vi "Main.vi"() -> ()   [LabVIEW 2019]
uses:
  <vilib>/myRIO/Instrument Drivers/Onboard IO/DIO/typedefs/DIO Reference.ctl
  <vilib>/myRIO/Common/Instrument Driver Framework/Utilities/typedefs/myRIO Generic Hardware Reference.ctl
  <vilib>/myRIO/Common/Instrument Driver Framework/Utilities/typedefs/Hardware Version Enum.ctl
  <vilib>/myRIO/Common/Instrument Driver Framework/Utilities/typedefs/myRIO v1.0 Reference.ctl
  <vilib>/myRIO/Common/Instrument Driver Framework/Utilities/typedefs/Generic FPGA Reference.ctl
  <vilib>/myRIO/Common/Instrument Driver Framework/myRIO v1.0/DIO/typedefs/DIO Channels List.ctl
  <vilib>/myRIO/Common/Instrument Driver Framework/myRIO v1.0/DIO/typedefs/DIO Channels Enum.ctl
  <vilib>/userDefined/High Color/nirio_resource_hc.ctl
  <vilib>/myRIO/Common/Instrument Driver Framework/myRIO v1.0/Encoder/typedefs/Encoder Signal Mode.ctl
  <vilib>/myRIO/Instrument Drivers/Onboard IO/Encoder/typedefs/Encoder Reference.ctl
  <vilib>/myRIO/Common/Instrument Driver Framework/myRIO v1.0/Encoder/typedefs/Encoder Channels Enum.ctl
  <vilib>/myRIO/Common/Instrument Driver Framework/myRIO v1.0/Encoder/typedefs/Encoder Configuration v1.0.ctl
  <vilib>/myRIO/Common/Instrument Driver Framework/Utilities/vis/Is FPGA Ref Available.vi
  <vilib>/myRIO/Common/Instrument Driver Framework/myRIO v1.0/DIO/vis/myRIO v1.1 Open DIO.vi
  <vilib>/myRIO/Instrument Drivers/Onboard IO/DIO/vis/Read.vi
  <vilib>/myRIO/Common/Instrument Driver Framework/myRIO v1.0/Encoder/vis/myRIO v1.1 Open Encoder.vi
  <vilib>/myRIO/Instrument Drivers/Onboard IO/Encoder/vis/Read.vi
  <vilib>/myRIO/Instrument Drivers/Onboard IO/DIO/vis/Write.vi
  <vilib>/myRIO/Common/Instrument Driver Framework/Utilities/vis/Validate Channels.vi
  <vilib>/myRIO/Common/Instrument Driver Framework/myRIO v1.0/DIO/vis/myRIO v1.0 Reserve DIO.vi
  <vilib>/myRIO/Common/Instrument Driver Framework/myRIO v1.0/Encoder/vis/myRIO v1.0 Reserve Encoder.vi
  <vilib>/Analysis/coordinate.llb/2D Cartesian Coordinate Rotation.vi
  <vilib>/Analysis/coordinate.llb/2D Cartesian Coordinate Rotation (Scalar).vi
  <vilib>/myRIO/Common/Instrument Driver Framework/myRIO v1.0/Resource Manager/vis/myRIO v1.0 Reserve Channel List.vi
  <vilib>/myRIO/Common/Instrument Driver Framework/myRIO v1.0/DIO/vis/myRIO v1.0 Build MUX Configuration DIO.vi
  <vilib>/myRIO/Common/Instrument Driver Framework/myRIO v1.0/Encoder/vis/myRIO v1.0 Build MUX Configuration Encoder.vi
  <vilib>/myRIO/Common/Instrument Driver Framework/myRIO v1.0/Resource Manager/vis/myRIO v1.0 Reserve Channel.vi
  <vilib>/myRIO/Common/Instrument Driver Framework/myRIO v1.0/Resource Manager/vis/myRIO v1.0 Unreserve Channel.vi
  <vilib>/myRIO/Common/Instrument Driver Framework/myRIO v1.0/Resource Manager/vis/myRIO v1.0 Create Configuration List.vi
  <vilib>/myRIO/Common/Instrument Driver Framework/myRIO v1.0/Resource Manager/vis/myRIO v1.0 Build Mutex Name.vi
  Global Var.vi
  <vilib>/Instr/_visa.llb/VISA Configure Serial Port (Instr).vi
  <vilib>/addons/control/pid/pid.llb/PID (DBL).vi
  <vilib>/Utility/VariantDataType/GetNumericInfo.vi
  <vilib>/Utility/error.llb/Error Cluster From Error Code.vi
  <vilib>/myRIO/Common/Instrument Driver Framework/myRIO v1.0/myRIO v1.1 Open.vi
  <vilib>/myRIO/Common/Instrument Driver Framework/Utilities/vis/IO Manager.vi
  <vilib>/myRIO/Common/Instrument Driver Framework/Utilities/vis/Configuration Manager.vi
  <vilib>/myRIO/Common/Instrument Driver Framework/myRIO v1.0/Resource Manager/vis/myRIO v1.0 Configure IO.vi
  <vilib>/myRIO/Common/Instrument Driver Framework/myRIO v1.0/myRIO v1.0 Close.vi
  <vilib>/myRIO/Common/Instrument Driver Framework/myRIO v1.0/DIO/vis/myRIO v1.0 Write DIO.vi
  <vilib>/myRIO/Common/Instrument Driver Framework/myRIO v1.0/Encoder/vis/myRIO v1.0 Configure Encoder.vi
  <vilib>/myRIO/Common/Instrument Driver Framework/myRIO v1.0/Encoder/vis/myRIO v1.0 Read Encoder.vi
  <vilib>/myRIO/Common/Instrument Driver Framework/myRIO v1.0/DIO/vis/myRIO v1.0 Read DIO.vi
  <vilib>/myRIO/Express VI/Onboard IO/DO/DO Express VI.xnode
  <vilib>/myRIO/Instrument Drivers/Onboard IO/DIO/vis/myRIO DIO Open.xnode
  <vilib>/myRIO/Express VI/Onboard IO/Encoder/Encoder Express VI.xnode
  <vilib>/myRIO/Instrument Drivers/Onboard IO/Encoder/vis/myRIO Encoder Open.xnode
  <vilib>/myRIO/Common/Instrument Driver Framework/myRIO v1.0/Encoder/typedefs/Encoder Count Direction Enum.ctl
  <vilib>/myRIO/Express VI/Onboard IO/DI/DI Express VI.xnode
  <vilib>/myRIO/Instrument Drivers/Onboard IO/DIO/DIO.lvlib
  <vilib>/myRIO/Instrument Drivers/Onboard IO/Encoder/Encoder.lvlib
  <vilib>/addons/control/pid/NI_PID_pid.lvlib
  <vilib>/robotics/Steering/Steering Frame/NI_Robotics_Steering Frame.lvclass
panel:
  in  "Reset":bool
  out "Suctime":u32
  out "lasttime":u32
  out "time":u32
  in  "QRCodeTick":bool
  out "read buffer":string
  in  "Set Y":dbl
  in  "Set 0":bool
  out "Chart Trackline 3":cluster{"X_set":dbl, "X_en":dbl}(graph)
  in  "PID gains 6":T1={"proportional gain (Kc)"=1.5, "integral time (Ti, min)"=0.0, "derivative time (Td, min)"=0.0} {"derivative time (Td, min)" format="%.3f"; "integral time (Ti, min)" format="%.3f"; "proportional gain (Kc)" format="%.3f"}
  in  "PID gains 5":T1={"proportional gain (Kc)"=1.0, "integral time (Ti, min)"=0.0, "derivative time (Td, min)"=0.0} {"derivative time (Td, min)" format="%.3f"; "integral time (Ti, min)" format="%.3f"; "proportional gain (Kc)" format="%.3f"}
  out "Chart Trackline 2":cluster{"X_set":dbl, "X_en":dbl}(graph)
  in  "PID gains 4":T1={"proportional gain (Kc)"=1.4, "integral time (Ti, min)"=0.0, "derivative time (Td, min)"=0.0} {"derivative time (Td, min)" format="%.3f"; "integral time (Ti, min)" format="%.3f"; "proportional gain (Kc)" format="%.3f"}
  out "Chart Trackline":cluster{"X_set":dbl, "X_en":dbl}(graph)
  out "Chart Theta":cluster{"X_set":dbl, "X_en":dbl}(graph)
  out "Chart Y":cluster{"X_set":dbl, "X_en":dbl}(graph)
  out "Chart X":cluster{"X_set":dbl, "X_en":dbl}(graph)
  out "OutTheta":dbl format="%.2f"
  in  "PID gains 3":T1={"proportional gain (Kc)"=3.0, "integral time (Ti, min)"=0.0, "derivative time (Td, min)"=0.0} {"derivative time (Td, min)" format="%.7f"; "integral time (Ti, min)" format="%.7f"; "proportional gain (Kc)" format="%.7f"}
  out "OutY":dbl format="%.2f"
  in  "PID gains 2":T1={"proportional gain (Kc)"=30.0, "integral time (Ti, min)"=0.0, "derivative time (Td, min)"=0.0} {"derivative time (Td, min)" format="%.7f"; "integral time (Ti, min)" format="%.7f"; "proportional gain (Kc)" format="%.7f"}
  in  "PID gains":T1={"proportional gain (Kc)"=30.0, "integral time (Ti, min)"=0.0, "derivative time (Td, min)"=0.0} {"derivative time (Td, min)" format="%.7f"; "integral time (Ti, min)" format="%.7f"; "proportional gain (Kc)" format="%.7f"}
  out "OutX":dbl format="%.2f"
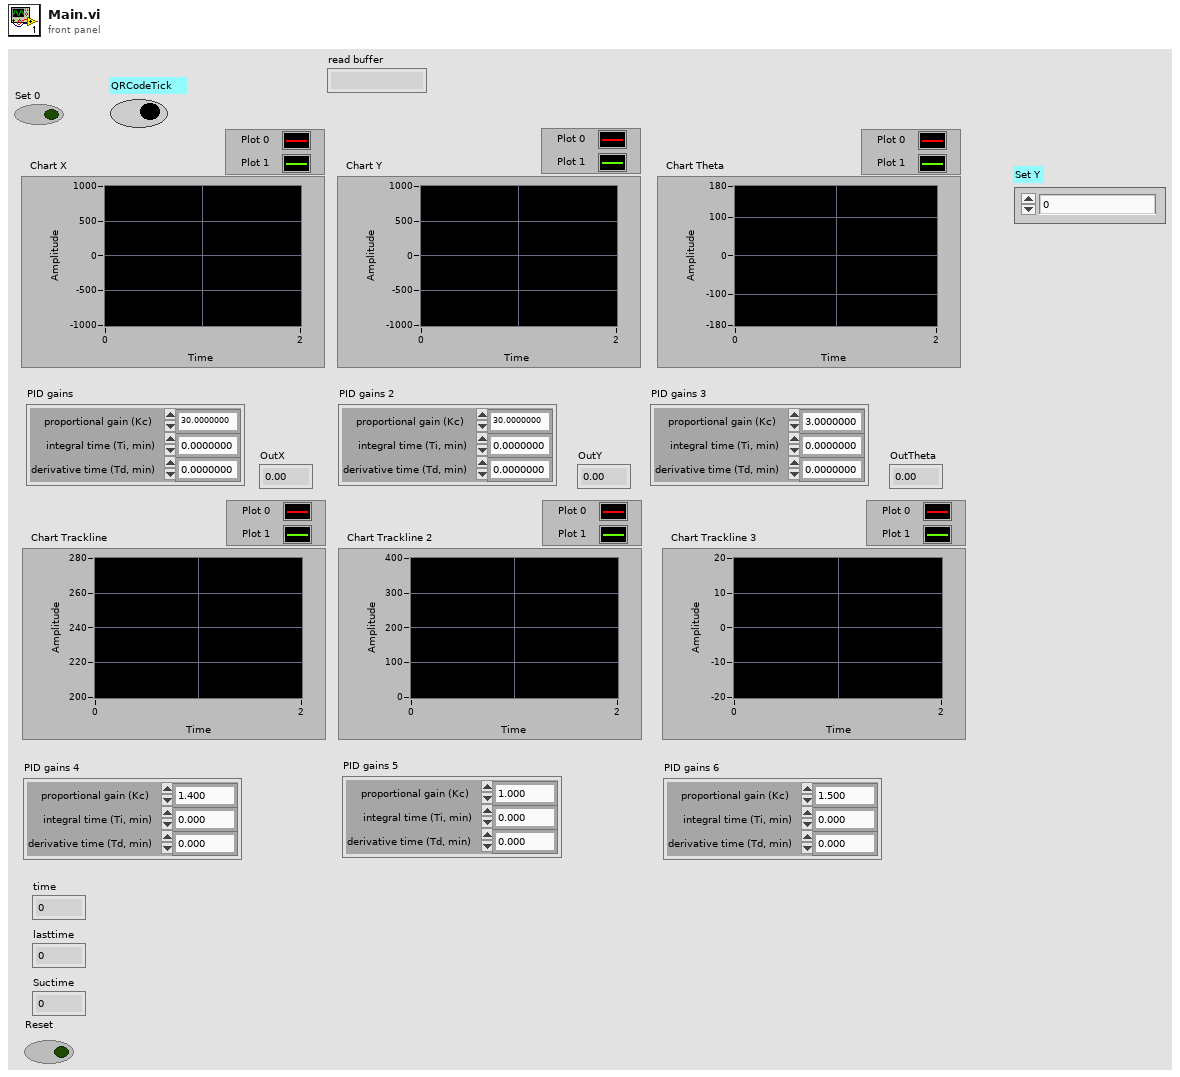
[diagram p1: front panel]
types:
  T1 = cluster{"proportional gain (Kc)":dbl, "integral time (Ti, min)":dbl, "derivative time (Td, min)":dbl}
  T2 = typedef "DIO.lvlib/DIO Reference.ctl" = cluster{"myRIO Reference":T3, "DIO Channels List":T7}
  T3 = typedef "myRIO Generic Hardware Reference.ctl" = cluster{"myRIO Model":T4, "myRIO Hardware Reference":T5}
  T4 = typedef "Hardware Version Enum.ctl" = enum16{"Unknown", "myRIO-1900", "myRIO-1950", "roboRIO", "NI ELVIS RIO CM", "ELVIS III"}
  T5 = typedef "myRIO v1.0 Reference.ctl" = cluster{"Generic FPGA Reference":T6, "Allow multiple opens":bool}
  T6 = typedef "Generic FPGA Reference.ctl" = refnum<k20>
  T7 = typedef "DIO Channels List.ctl" = T8[]
  T8 = typedef "DIO Channels Enum.ctl" = enum16{"Not Connected", "C/DIO0", "C/DIO1", "C/DIO2", "C/DIO3", "C/DIO4", "C/DIO5", "C/DIO6", "C/DIO7", "A/DIO0", "A/DIO1", "A/DIO2", "A/DIO3", "A/DIO4", "A/DIO5", "A/DIO6", "A/DIO7", "A/DIO8", "A/DIO9", "A/DIO10", "A/DIO11", "A/DIO12", "A/DIO13", "A/DIO14", "A/DIO15", "A/DIO16", "A/DIO17", "A/DIO18", "A/DIO19", "B/DIO0", "B/DIO1", "B/DIO2", "B/DIO3", "B/DIO4", "B/DIO5", "B/DIO6", "B/DIO7", "B/DIO8", "B/DIO9", "B/DIO10", "B/DIO11", "B/DIO12", "B/DIO13", "B/DIO14", "B/DIO15", "B/DIO16", "B/DIO17", "B/DIO18", "B/DIO19", "LED0", "LED1", "LED2", "LED3", "Button0", "DIO/DIO0", "DIO/DIO1", "DIO/DIO2", "DIO/DIO3", "DIO/DIO4", "DIO/DIO5", "DIO/DIO6", "DIO/DIO7", "DIO/DIO8", "DIO/DIO9", "SPI/CS0", "SPI/CS1", "SPI/CS2", "SPI/CS3", "LED RADIO (Green)", "LED RADIO (Red)", "LED COMM (Green)", "LED COMM (Red)", "LED MODE (Green)", "LED MODE (Red)"}
  T9 = typedef "nirio_resource_hc.ctl" = tag
  T10 = typedef "Encoder.lvlib/Encoder Reference.ctl" = cluster{"myRIO Reference":T3, "Encoder Channels Enum":T11}
  T11 = typedef "Encoder Channels Enum.ctl" = enum16{"Not Connected", "C/ENC0", "C/ENC1", "A/ENC", "A/ENC0", "A/ENC1", "A/ENC2", "A/ENC3", "A/ENC4", "A/ENC5", "A/ENC6", "A/ENC7", "A/ENC8", "A/ENC9", "B/ENC", "B/ENC0", "B/ENC1", "B/ENC2", "B/ENC3", "B/ENC4", "B/ENC5", "B/ENC6", "B/ENC7", "B/ENC8", "B/ENC9", "DIO/ENC0", "DIO/ENC1", "DIO/ENC2", "DIO/ENC3", "DIO/ENC4"}
  T12 = typedef "Encoder Signal Mode.ctl" = enum16{"Quadrature phase signal", "Step and direction signal"}
  T13 = cluster{"Cross set":dbl, "Cross Line Position":dbl}
  T14 = typedef "IMAQ Image.ctl" = refnum<image>
  T15 = cluster{"Point1 (Pixels)":cluster{"X":sgl, "Y":sgl}, "Point2 (Pixels)":cluster{"X":sgl, "Y":sgl}, "Point1 (Real-World)":cluster{"X":sgl, "Y":sgl}, "Point2 (Real-World)":cluster{"X":sgl, "Y":sgl}, "Angle (Pixel)":dbl, "Angle (Real-World)":dbl, "Score":dbl, "Straightness":dbl, "Average SNR (db)":dbl, "Calibration Valid":bool}
  T16 = cluster{"Point1 (Pixels)":cluster{"X":sgl, "Y":sgl}, "Point2 (Pixels)":cluster{"X":sgl, "Y":sgl}, "Point1 (Real-World)":cluster{"X":sgl, "Y":sgl}, "Point2 (Real-World)":cluster{"X":sgl, "Y":sgl}, "Angle (Pixel)":dbl, "Angle (Real-World)":dbl, "Score":dbl, "Straightness":dbl, "Average SNR (db)":dbl, "Calibration Valid":bool}[]
  T17 = cluster{"Straight Edges (Adv. Straight Edge 1)[0]":cluster{"Point1 (Pixels)":cluster{"X":sgl, "Y":sgl}, "Point2 (Pixels)":cluster{"X":sgl, "Y":sgl}, "Point1 (Real-World)":cluster{"X":sgl, "Y":sgl}, "Point2 (Real-World)":cluster{"X":sgl, "Y":sgl}, "Angle (Pixel)":dbl, "Angle (Real-World)":dbl, "Score":dbl, "Straightness":dbl, "Average SNR (db)":dbl, "Calibration Valid":bool}, "Straight Edges (Adv. Straight Edge 1)[1]":cluster{"Point1 (Pixels)":cluster{"X":sgl, "Y":sgl}, "Point2 (Pixels)":cluster{"X":sgl, "Y":sgl}, "Point1 (Real-World)":cluster{"X":sgl, "Y":sgl}, "Point2 (Real-World)":cluster{"X":sgl, "Y":sgl}, "Angle (Pixel)":dbl, "Angle (Real-World)":dbl, "Score":dbl, "Straightness":dbl, "Average SNR (db)":dbl, "Calibration Valid":bool}, "Straight Edges (Adv. Straight Edge 1)[2]":cluster{"Point1 (Pixels)":cluster{"X":sgl, "Y":sgl}, "Point2 (Pixels)":cluster{"X":sgl, "Y":sgl}, "Point1 (Real-World)":cluster{"X":sgl, "Y":sgl}, "Point2 (Real-World)":cluster{"X":sgl, "Y":sgl}, "Angle (Pixel)":dbl, "Angle (Real-World)":dbl, "Score":dbl, "Straightness":dbl, "Average SNR (db)":dbl, "Calibration Valid":bool}, "Straight Edges (Adv. Straight Edge 1)[3]":cluster{"Point1 (Pixels)":cluster{"X":sgl, "Y":sgl}, "Point2 (Pixels)":cluster{"X":sgl, "Y":sgl}, "Point1 (Real-World)":cluster{"X":sgl, "Y":sgl}, "Point2 (Real-World)":cluster{"X":sgl, "Y":sgl}, "Angle (Pixel)":dbl, "Angle (Real-World)":dbl, "Score":dbl, "Straightness":dbl, "Average SNR (db)":dbl, "Calibration Valid":bool}, "Straight Edges (Adv. Straight Edge 1)[4]":cluster{"Point1 (Pixels)":cluster{"X":sgl, "Y":sgl}, "Point2 (Pixels)":cluster{"X":sgl, "Y":sgl}, "Point1 (Real-World)":cluster{"X":sgl, "Y":sgl}, "Point2 (Real-World)":cluster{"X":sgl, "Y":sgl}, "Angle (Pixel)":dbl, "Angle (Real-World)":dbl, "Score":dbl, "Straightness":dbl, "Average SNR (db)":dbl, "Calibration Valid":bool}, "Straight Edges (Adv. Straight Edge 1)[5]":cluster{"Point1 (Pixels)":cluster{"X":sgl, "Y":sgl}, "Point2 (Pixels)":cluster{"X":sgl, "Y":sgl}, "Point1 (Real-World)":cluster{"X":sgl, "Y":sgl}, "Point2 (Real-World)":cluster{"X":sgl, "Y":sgl}, "Angle (Pixel)":dbl, "Angle (Real-World)":dbl, "Score":dbl, "Straightness":dbl, "Average SNR (db)":dbl, "Calibration Valid":bool}, "Straight Edges (Adv. Straight Edge 1)[6]":cluster{"Point1 (Pixels)":cluster{"X":sgl, "Y":sgl}, "Point2 (Pixels)":cluster{"X":sgl, "Y":sgl}, "Point1 (Real-World)":cluster{"X":sgl, "Y":sgl}, "Point2 (Real-World)":cluster{"X":sgl, "Y":sgl}, "Angle (Pixel)":dbl, "Angle (Real-World)":dbl, "Score":dbl, "Straightness":dbl, "Average SNR (db)":dbl, "Calibration Valid":bool}, "Straight Edges (Adv. Straight Edge 1)[7]":cluster{"Point1 (Pixels)":cluster{"X":sgl, "Y":sgl}, "Point2 (Pixels)":cluster{"X":sgl, "Y":sgl}, "Point1 (Real-World)":cluster{"X":sgl, "Y":sgl}, "Point2 (Real-World)":cluster{"X":sgl, "Y":sgl}, "Angle (Pixel)":dbl, "Angle (Real-World)":dbl, "Score":dbl, "Straightness":dbl, "Average SNR (db)":dbl, "Calibration Valid":bool}, "Straight Edges (Adv. Straight Edge 1)[8]":cluster{"Point1 (Pixels)":cluster{"X":sgl, "Y":sgl}, "Point2 (Pixels)":cluster{"X":sgl, "Y":sgl}, "Point1 (Real-World)":cluster{"X":sgl, "Y":sgl}, "Point2 (Real-World)":cluster{"X":sgl, "Y":sgl}, "Angle (Pixel)":dbl, "Angle (Real-World)":dbl, "Score":dbl, "Straightness":dbl, "Average SNR (db)":dbl, "Calibration Valid":bool}}
  T18 = cluster{"Straight Edges (Adv. Straight Edge 3)[0]":cluster{"Point1 (Pixels)":cluster{"X":sgl, "Y":sgl}, "Point2 (Pixels)":cluster{"X":sgl, "Y":sgl}, "Point1 (Real-World)":cluster{"X":sgl, "Y":sgl}, "Point2 (Real-World)":cluster{"X":sgl, "Y":sgl}, "Angle (Pixel)":dbl, "Angle (Real-World)":dbl, "Score":dbl, "Straightness":dbl, "Average SNR (db)":dbl, "Calibration Valid":bool}, "Straight Edges (Adv. Straight Edge 3)[1]":cluster{"Point1 (Pixels)":cluster{"X":sgl, "Y":sgl}, "Point2 (Pixels)":cluster{"X":sgl, "Y":sgl}, "Point1 (Real-World)":cluster{"X":sgl, "Y":sgl}, "Point2 (Real-World)":cluster{"X":sgl, "Y":sgl}, "Angle (Pixel)":dbl, "Angle (Real-World)":dbl, "Score":dbl, "Straightness":dbl, "Average SNR (db)":dbl, "Calibration Valid":bool}, "Straight Edges (Adv. Straight Edge 3)[2]":cluster{"Point1 (Pixels)":cluster{"X":sgl, "Y":sgl}, "Point2 (Pixels)":cluster{"X":sgl, "Y":sgl}, "Point1 (Real-World)":cluster{"X":sgl, "Y":sgl}, "Point2 (Real-World)":cluster{"X":sgl, "Y":sgl}, "Angle (Pixel)":dbl, "Angle (Real-World)":dbl, "Score":dbl, "Straightness":dbl, "Average SNR (db)":dbl, "Calibration Valid":bool}, "Straight Edges (Adv. Straight Edge 3)[3]":cluster{"Point1 (Pixels)":cluster{"X":sgl, "Y":sgl}, "Point2 (Pixels)":cluster{"X":sgl, "Y":sgl}, "Point1 (Real-World)":cluster{"X":sgl, "Y":sgl}, "Point2 (Real-World)":cluster{"X":sgl, "Y":sgl}, "Angle (Pixel)":dbl, "Angle (Real-World)":dbl, "Score":dbl, "Straightness":dbl, "Average SNR (db)":dbl, "Calibration Valid":bool}, "Straight Edges (Adv. Straight Edge 3)[4]":cluster{"Point1 (Pixels)":cluster{"X":sgl, "Y":sgl}, "Point2 (Pixels)":cluster{"X":sgl, "Y":sgl}, "Point1 (Real-World)":cluster{"X":sgl, "Y":sgl}, "Point2 (Real-World)":cluster{"X":sgl, "Y":sgl}, "Angle (Pixel)":dbl, "Angle (Real-World)":dbl, "Score":dbl, "Straightness":dbl, "Average SNR (db)":dbl, "Calibration Valid":bool}, "Straight Edges (Adv. Straight Edge 3)[5]":cluster{"Point1 (Pixels)":cluster{"X":sgl, "Y":sgl}, "Point2 (Pixels)":cluster{"X":sgl, "Y":sgl}, "Point1 (Real-World)":cluster{"X":sgl, "Y":sgl}, "Point2 (Real-World)":cluster{"X":sgl, "Y":sgl}, "Angle (Pixel)":dbl, "Angle (Real-World)":dbl, "Score":dbl, "Straightness":dbl, "Average SNR (db)":dbl, "Calibration Valid":bool}, "Straight Edges (Adv. Straight Edge 3)[6]":cluster{"Point1 (Pixels)":cluster{"X":sgl, "Y":sgl}, "Point2 (Pixels)":cluster{"X":sgl, "Y":sgl}, "Point1 (Real-World)":cluster{"X":sgl, "Y":sgl}, "Point2 (Real-World)":cluster{"X":sgl, "Y":sgl}, "Angle (Pixel)":dbl, "Angle (Real-World)":dbl, "Score":dbl, "Straightness":dbl, "Average SNR (db)":dbl, "Calibration Valid":bool}, "Straight Edges (Adv. Straight Edge 3)[7]":cluster{"Point1 (Pixels)":cluster{"X":sgl, "Y":sgl}, "Point2 (Pixels)":cluster{"X":sgl, "Y":sgl}, "Point1 (Real-World)":cluster{"X":sgl, "Y":sgl}, "Point2 (Real-World)":cluster{"X":sgl, "Y":sgl}, "Angle (Pixel)":dbl, "Angle (Real-World)":dbl, "Score":dbl, "Straightness":dbl, "Average SNR (db)":dbl, "Calibration Valid":bool}, "Straight Edges (Adv. Straight Edge 3)[8]":cluster{"Point1 (Pixels)":cluster{"X":sgl, "Y":sgl}, "Point2 (Pixels)":cluster{"X":sgl, "Y":sgl}, "Point1 (Real-World)":cluster{"X":sgl, "Y":sgl}, "Point2 (Real-World)":cluster{"X":sgl, "Y":sgl}, "Angle (Pixel)":dbl, "Angle (Real-World)":dbl, "Score":dbl, "Straightness":dbl, "Average SNR (db)":dbl, "Calibration Valid":bool}}
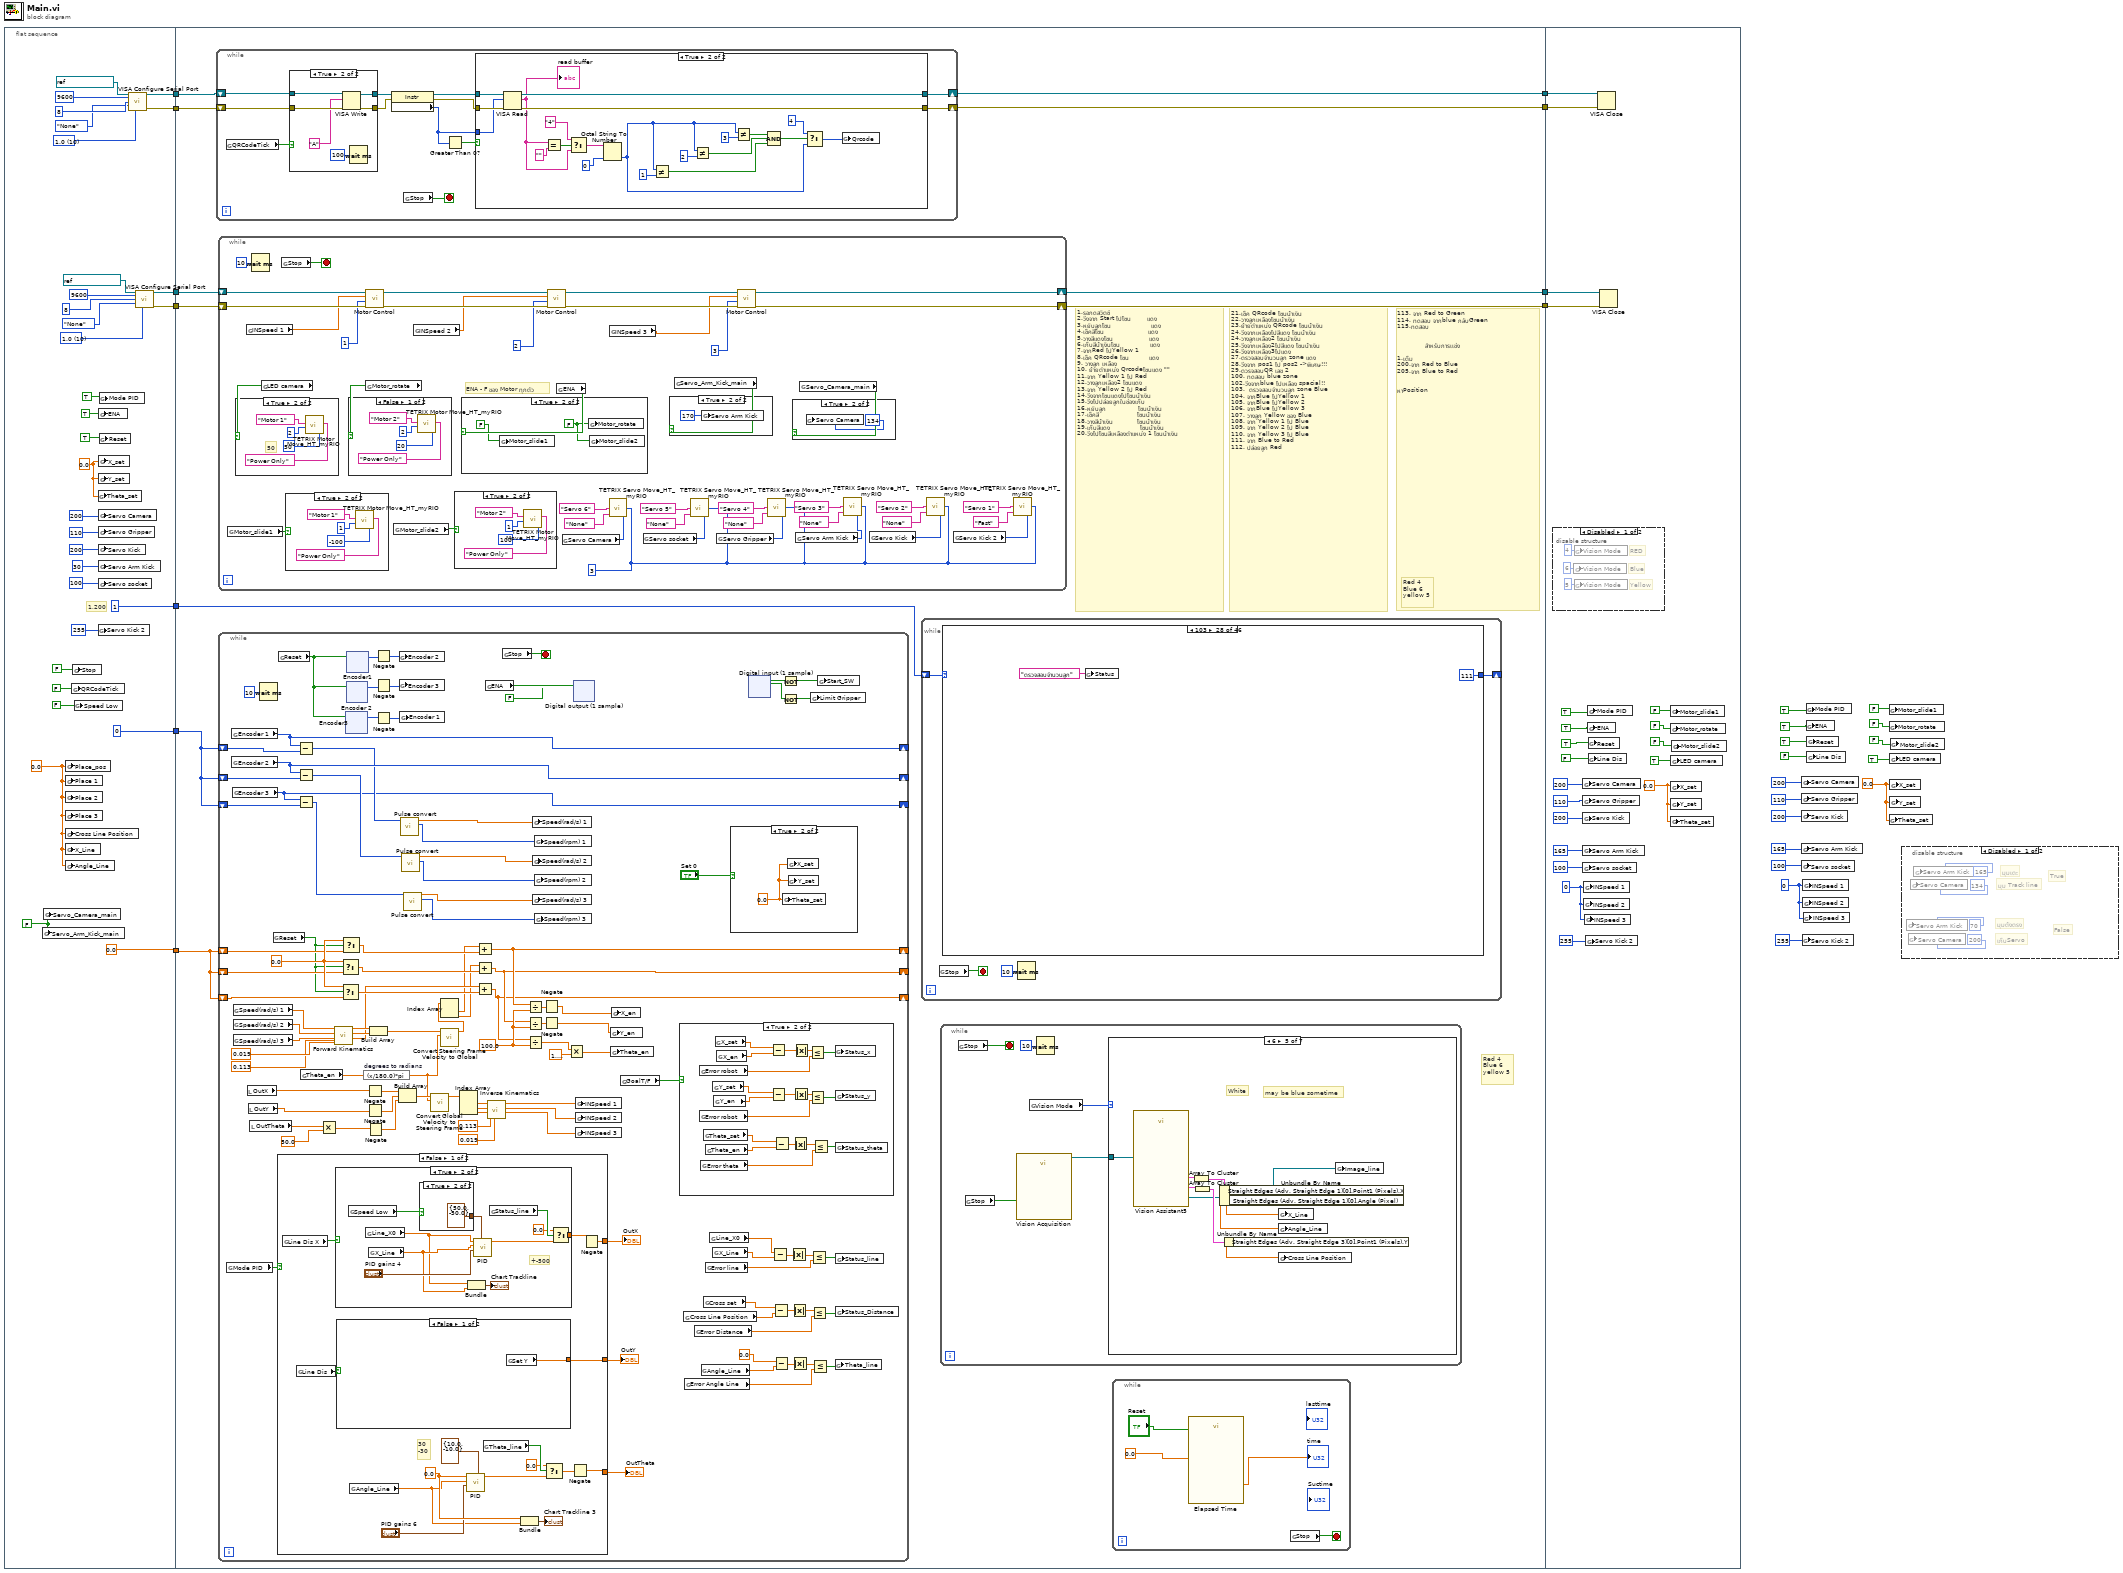
[diagram p0: block diagram]
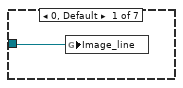
[diagram p3: hidden frame]
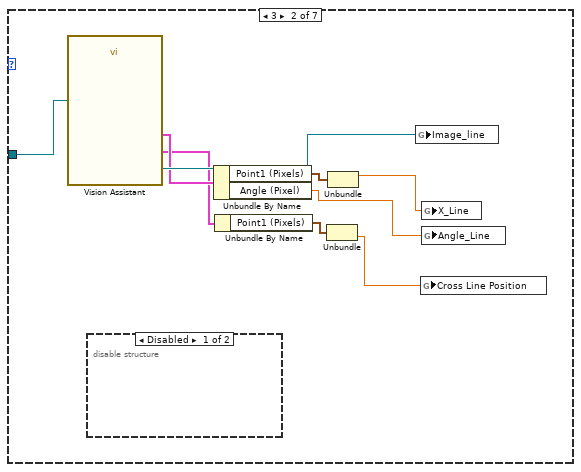
[diagram p4: hidden frame]
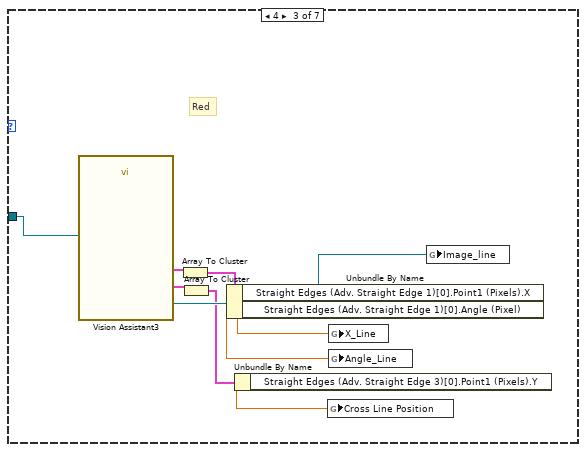
[diagram p6: hidden frame]
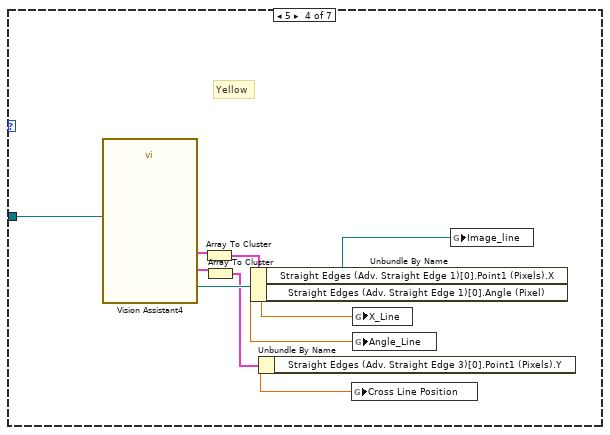
[diagram p7: hidden frame]
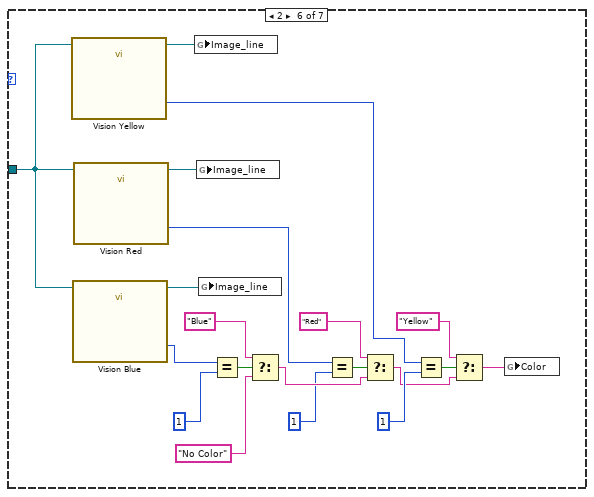
[diagram p8: hidden frame]
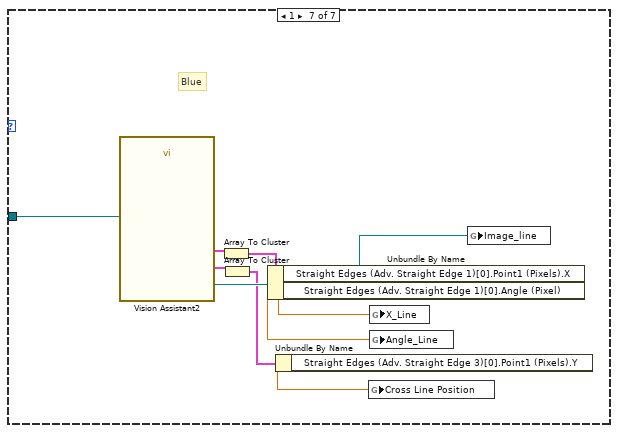
[diagram p9: hidden frame]
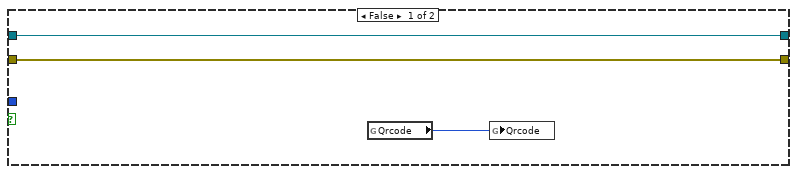
[diagram p10: hidden frame]
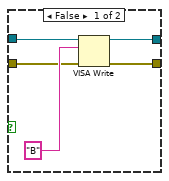
[diagram p11: hidden frame]
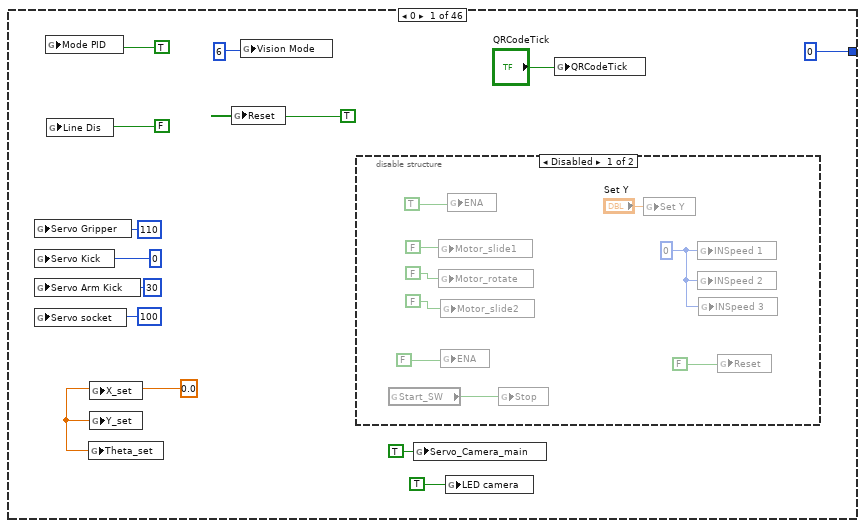
[diagram p12: hidden frame]
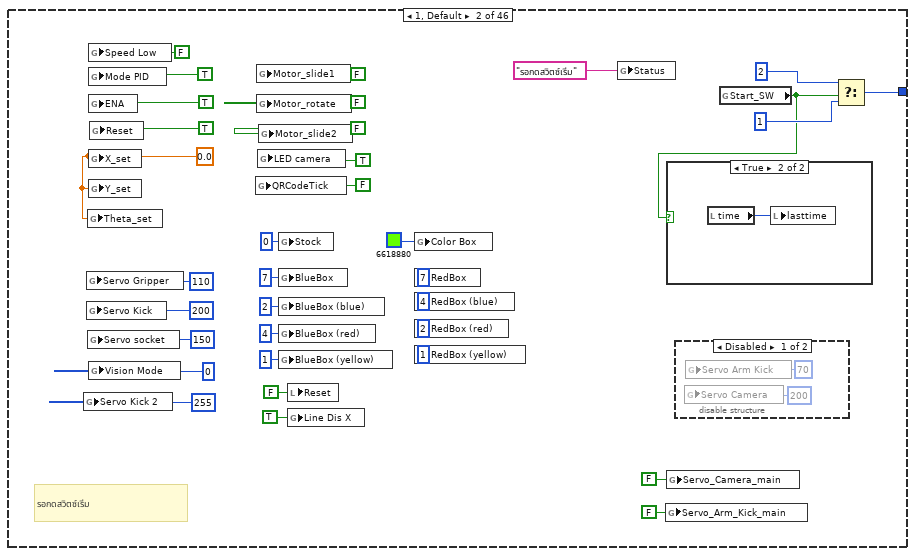
[diagram p14: hidden frame]
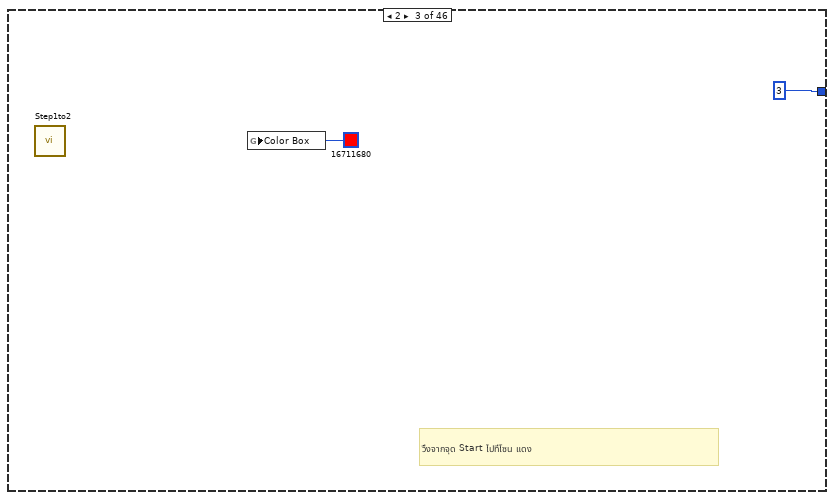
[diagram p17: hidden frame]
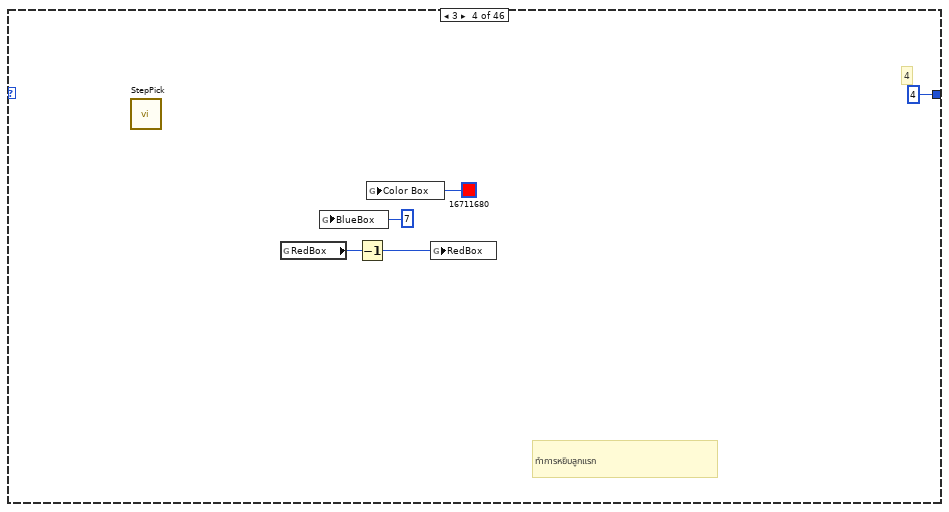
[diagram p18: hidden frame]
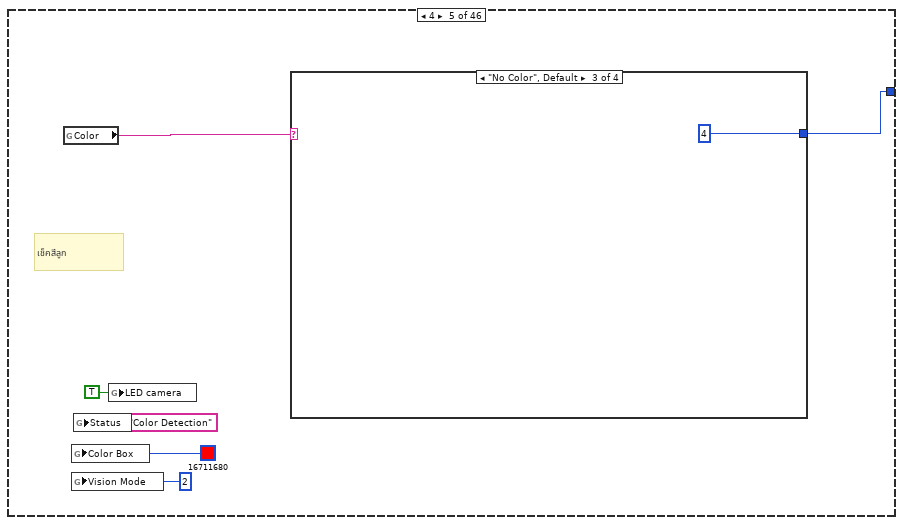
[diagram p19: hidden frame]
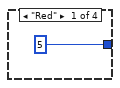
[diagram p20: hidden frame]
diagram:
  w10 = i16 0 ("INSpeed 1")
  w11 = 0.0 ("X_set")
  n1 = flat-sequence {
    tunnel: [0.0 ("t")] -> w27
    tunnel: [0] -> w26
    tunnel: [1] -> w25
    tunnel: [w40] -> w8
    tunnel: [w39] -> w7
    tunnel: [w32] -> w2
    tunnel: [w31] -> w1
    tunnel: w27 -> [w70]
    tunnel: w26 -> [w69]
    tunnel: w25 -> [w68]
    tunnel: w8 -> [w67]
    tunnel: w7 -> [w66]
    tunnel: [w65] -> w6
    tunnel: [w64] -> w5
    tunnel: [w63] -> w4
    tunnel: [w62] -> w3
    tunnel: w2 -> [w61]
    tunnel: w1 -> [w60]
    tunnel: w6 -> [w1206]
    tunnel: w5 -> [w1205]
    tunnel: w4 -> [w1204]
    tunnel: w3 -> [w1203]
    frame #0 {
      w28 = FALSE ("Mode PID")
      w30 = 0.0 ("Place_pos")
      w33 = u16 10 items=["1.0"=10, "1.5"=15, "2.0"=20] ("stop bits (10: 1 bit)")
      w43 = u16 10 items=["1.0"=10, "1.5"=15, "2.0"=20] ("stop bits (10: 1 bit)")
      w58 = 0.0 ("X_set")
      # "1,200"
      n2 = global write "Global Var.vi" "Servo_Arm_Kick_main"(w28) -> ()
      n3 = global write "Global Var.vi" "Servo_Camera_main"(w28) -> ()
      n4 = global write "Global Var.vi" "Place_pos"(w30) -> ()
      n5 = global write "Global Var.vi" "Place 1"(w30) -> ()
      n6 = global write "Global Var.vi" "Place 2"(w30) -> ()
      n7 = global write "Global Var.vi" "Place 3"(w30) -> ()
      n8 = global write "Global Var.vi" "Cross Line Position"(w30) -> ()
      n9 = global write "Global Var.vi" "X_Line"(w30) -> ()
      n10 = global write "Global Var.vi" "Angle_Line"(w30) -> ()
      n11 = global write "Global Var.vi" "QRCodeTick"(FALSE ("Mode PID")) -> ()
      n12 = global write "Global Var.vi" "Stop"(FALSE ("ENA")) -> ()
      n13 = global write "Global Var.vi" "Speed Low"(FALSE ("Mode PID")) -> ()
      n14 = global write "Global Var.vi" "Theta_set"(w58) -> ()
      n15 = global write "Global Var.vi" "Servo Kick 2"(u8 255 ("Servo Camera")) -> ()
      n16 = global write "Global Var.vi" "ENA"(TRUE ("ENA")) -> ()
      n17 = global write "Global Var.vi" "X_set"(w58) -> ()
      n18 = global write "Global Var.vi" "Y_set"(w58) -> ()
      n19 = global write "Global Var.vi" "Servo Camera"(u8 200 ("Servo Camera")) -> ()
      n20 = global write "Global Var.vi" "Servo Gripper"(u8 110 ("Servo Camera")) -> ()
      n21 = global write "Global Var.vi" "Servo Kick"(u8 200 ("Servo Camera")) -> ()
      n22 = global write "Global Var.vi" "Servo Arm Kick"(u8 30 ("Servo Camera")) -> ()
      n23 = global write "Global Var.vi" "Servo socket"(u8 100 ("Servo Camera")) -> ()
      n24 = global write "Global Var.vi" "Mode PID"(TRUE ("Mode PID")) -> ()
      n25 = global write "Global Var.vi" "Reset"(TRUE ("ENA")) -> ()
      n26 = call-poly "VISA Configure Serial Port"("VISA resource name"=refnum<visa-resource-name> "ASRL1::INSTR", "baud rate (9600)"=u32 9600, "data bits (8)"=u16 8, "parity (0:none)"=enum16{"None", "Odd", "Even", "Mark", "Space"}."None", "stop bits (10: 1 bit)"=w33) -> ("VISA resource name out"=w32:refnum<visa-resource-name>, "error out"=w31:errorcluster)  [unwired: 9 in]
      n27 = call-poly "VISA Configure Serial Port"("VISA resource name"=refnum<visa-resource-name> "ASRL2::INSTR", "baud rate (9600)"=u32 9600, "data bits (8)"=u16 8, "parity (0:none)"=enum16{"None", "Odd", "Even", "Mark", "Space"}."None", "stop bits (10: 1 bit)"=w43) -> ("VISA resource name out"=w40:refnum<visa-resource-name>, "error out"=w39:errorcluster)  [unwired: 9 in]
    }
    frame #1 {
      # "Red 4\nBlue 6\nyellow 5"
      # "Red 4\nBlue 6\nyellow 5"
      # "113. จาก Red to Green\n114. ทดสอบ จากblue กลับGreen\n115.ทดสอบ\n\n\n              สำหรับการเเข่ง\n\n1.เต็ม\n200.จาก Red to Blue\n205.จาก Blue to Red\n\n\nหาPosition"
      # "21.เช็ค QRcode โซนน้ำเงิน\n22.วางลูกเหลืองโซนน้ำเงิน\n23.ย้ายตำแหน่ง QRcode โซนน้ำเงิน\n24.วิ่งจากเหลืองไปสีแดง โซนน้ำเงิน\n24.วางลูกเหลือง2 โซนน้ำเงิน\n25.วิ่งจากเหลือง2ไปสีแดง โซนน้ำเงิน\n26.วิ่งจากเหลือง3ไปแดง\n27.ตรวจสอบจำนวนลูก zone แดง\n28.วิ่งจาก pos1 ไป pos2 ->พิเศษ!!!\n29.ตวรจสอบQR เลข 2  \n100. ทดสอบ blue zone   \n102.วิ่งจากblue ไปเหลือง spacial!!\n103.  ตรวจสอบจำนวนลูก zone Blue\n104. จากBlue ไปYellow 1\n105. จากBlue ไปYellow 2\n106. จากBlue ไปYellow 3\n107. วางลูก Yellow ของ Blue\n108. จาก Yellow 1 ไป Blue\n109. จาก Yellow 2 ไป Blue\n110. จาก Yellow 3 ไป Blue\n111. จาก Blue to Red \n112. ปล่อยลูก Red"
      # "1.รอกดสวิตซ์\n2.วิ่งจาก Start ไปโซน        แดง\n3.หยิบลูกโซน                    แดง\n4.เช็คสีโซน                      แดง\n5.วางสีแดงโซน                  แดง\n6.เก็บสีน้ำเงินโซน               แดง\n7.จากRed ไปYellow 1\n8.เช็ค QRcode โซน          แดง\n9. วางลูก เหลือง\n10. ย้ายตำแหน่ง Qrcodeโซนแดง \"\"\n11.จาก Yellow 1 ไป Red\n12.วางลูกเหลือง2 โซนแดง\n13.จาก Yellow 2 ไป Red \n14.วิ่งจากโซนแดงไปโซนน้ำเงิน\n15.วิ่งไปปล่อยลูกในช่องเก็บ\n16.หยิบลูก                โซนน้ำเงิน\n17.เช็คสี                   โซนน้ำเงิน\n18.วางสีน้ำเงิน            โซนน้ำเงิน\n19.เก็บสีแดง               โซนน้ำเงิน\n20.วิ่งไปโซนสีเหลืองตำแหน่ง 1 โซนน้ำเงิน"
      n28 = while {
        shift-right: [w156] -> w63
        shift-left: w60 -> [w152]
        shift-right: [w157] -> w62
        shift-left: w61 -> [w153]
        stop <- w155 stop-if-true
        n29 = global read "Global Var.vi" "QRCodeTick"() -> (w154:bool)
        n30 = case shown="True" w154 {
          tunnel: w153 -> [w185 w192]
          tunnel: w152 -> [w184 w191]
          tunnel: [w182 w189] -> w151
          tunnel: [w183 w188] -> w150
          frame False {
            n31 = VISA Write(VISA resource name=w185, write buffer="B", error in (no error)=w184) -> (VISA resource name out=w182:refnum<visa-resource-name>, error out=w183:errorcluster)  [unwired: 1 out]
          }
          frame True {
            n32 = VISA Write(VISA resource name=w192, write buffer="A", error in (no error)=w191) -> (VISA resource name out=w189:refnum<visa-resource-name>, error out=w188:errorcluster)  [unwired: 1 out]
            n33 = Wait (ms)(milliseconds to wait=u32 100) -> ()  [unwired: 1 out]
          }
        }
        n34 = property class="Instr"(reference=w151, error in=w150) -> (reference out=w148:refnum<visa-resource-name>, error out=w147:errorcluster, "Serial Settings:Number of Bytes at Serial Port"=w146:u32)
        n35 = global read "Global Var.vi" "Stop"() -> (w155:bool)
        n36 = Greater Than 0?(x=w146) -> (x > 0?=w149:bool)
        n37 = case shown="True" w149 {
          tunnel: [w160 w181] -> w157
          tunnel: [w159 w180] -> w156
          tunnel: w148 -> [w160 w179]
          tunnel: w147 -> [w159 w178]
          tunnel: w146 -> [_ w177]
          frame False {
            n38 = global read "Global Var.vi" "Qrcode"() -> (w158:i16)
            n39 = global write "Global Var.vi" "Qrcode"(w158) -> ()
          }
          frame True {
            n40 = VISA Read(VISA resource name=w179, byte count=w177, error in (no error)=w178) -> (VISA resource name out=w181:refnum<visa-resource-name>, read buffer=w171:string, error out=w180:errorcluster)  [unwired: 1 out]
            "read buffer" <- w171
            n41 = Equal?(x=w171, y="") -> (x = y?=w175:bool)
            n42 = Select(t="4", s=w175, f=w171) -> (s? t:f=w173:string)
            n43 = Octal String To Number(2:i16 0, 4:w173) -> (0:w162:i16)  [unwired: 1 in, 1 out]
            n44 = Not Equal?(x=w162, y=i16 1) -> (x != y?=w165:bool)
            n45 = Not Equal?(x=w162, y=i16 2) -> (x != y?=w166:bool)
            n46 = Not Equal?(x=w162, y=i16 3) -> (x != y?=w167:bool)
            n47 = Compound Arithmetic op=AND(w167, w166, w165) -> (w164:bool)
            n48 = Select(t=i16 4 ("y"), s=w164, f=w162) -> (s? t:f=w161:i16)
            n49 = global write "Global Var.vi" "Qrcode"(w161) -> ()
          }
        }
      }
      n50 = while {
        shift-right: [w1132] -> w65
        shift-left: w67 -> [w1138]
        shift-right: [w1131] -> w64
        shift-left: w66 -> [w1137]
        stop <- w1153 stop-if-true
        w1139 = u8 3 ("Controller Daisy Chain Position (1 - 4)")
        # "ENA - F ของ Motor ทุกตัว"
        n51 = global read "Global Var.vi" "Motor_slide1"() -> (w1150:bool)
        n52 = global read "Global Var.vi" "INSpeed 1"() -> (w1125:dbl)
        n53 = Wait (ms)(milliseconds to wait=u32 10) -> ()  [unwired: 1 out]
        n54 = global read "Global Var.vi" "LED camera"() -> (w1151:bool)
        n55 = case shown="True" w1151 {
          frame False {
            n56 = call <vilib>:"TETRIX Motor Move_HT_myRIO.vi"("Power (-100 to 100)\n0 = Stop/Brake\n-128 = Stop/Coast"=i8 0 ("Power (-100 to 100)\n0 = Stop/Brake\n-128 = Stop/Coast"), "Control Mode"="Power Only", "Controller Daisy Chain Position: 1 - 4"=u8 2, "Select Channel"="Motor 1") -> ()  [unwired: 3 in, 1 out]
          }
          frame True {
            # "50"
            n57 = call <vilib>:"TETRIX Motor Move_HT_myRIO.vi"("Power (-100 to 100)\n0 = Stop/Brake\n-128 = Stop/Coast"=50 ("Encoder Target: 360 = 1 motor shaft revolution"), "Control Mode"="Power Only", "Controller Daisy Chain Position: 1 - 4"=u8 2, "Select Channel"="Motor 1") -> ()  [unwired: 3 in, 1 out]
          }
        }
        n58 = global read "Global Var.vi" "Stop"() -> (w1153:bool)
        n59 = case shown="True" w1150 {
          frame False {
            n60 = call <vilib>:"TETRIX Motor Move_HT_myRIO.vi"("Power (-100 to 100)\n0 = Stop/Brake\n-128 = Stop/Coast"=i8 60 ("Power (-100 to 100)\n0 = Stop/Brake\n-128 = Stop/Coast"), "Control Mode"="Power Only", "Controller Daisy Chain Position: 1 - 4"=u8 1, "Select Channel"="Motor 1") -> ()  [unwired: 3 in, 1 out]
          }
          frame True {
            n61 = call <vilib>:"TETRIX Motor Move_HT_myRIO.vi"("Power (-100 to 100)\n0 = Stop/Brake\n-128 = Stop/Coast"=-100 ("Encoder Target: 360 = 1 motor shaft revolution"), "Control Mode"="Power Only", "Controller Daisy Chain Position: 1 - 4"=u8 1, "Select Channel"="Motor 1") -> ()  [unwired: 3 in, 1 out]
          }
        }
        n62 = call "Motor Control.vi"("error in (no error)"=w1137, "MotorSelect"=i16 1, "INSpeed"=w1125, "VISA Refnum in"=w1138) -> ("error out"=w1135:errorcluster, "VISA Refnum out"=w1136:refnum<visa-resource-name>)  [unwired: 6 in]
        n63 = global read "Global Var.vi" "Motor_rotate"() -> (w1149:bool)
        n64 = case shown="False" w1149 {
          frame False {
            n65 = call <vilib>:"TETRIX Motor Move_HT_myRIO.vi"("Power (-100 to 100)\n0 = Stop/Brake\n-128 = Stop/Coast"=i8 20 ("Power (-100 to 100)\n0 = Stop/Brake\n-128 = Stop/Coast"), "Control Mode"="Power Only", "Controller Daisy Chain Position: 1 - 4"=u8 2, "Select Channel"="Motor 2") -> ()  [unwired: 3 in, 1 out]
          }
          frame True {
            n66 = call <vilib>:"TETRIX Motor Move_HT_myRIO.vi"("Power (-100 to 100)\n0 = Stop/Brake\n-128 = Stop/Coast"=-20 ("Encoder Target: 360 = 1 motor shaft revolution"), "Control Mode"="Power Only", "Controller Daisy Chain Position: 1 - 4"=u8 2, "Select Channel"="Motor 2") -> ()  [unwired: 3 in, 1 out]
          }
        }
        n67 = global read "Global Var.vi" "Motor_slide2"() -> (w1148:bool)
        n68 = global read "Global Var.vi" "INSpeed 2"() -> (w1126:dbl)
        n69 = case shown="True" w1148 {
          frame False {
            n70 = call <vilib>:"TETRIX Motor Move_HT_myRIO.vi"("Power (-100 to 100)\n0 = Stop/Brake\n-128 = Stop/Coast"=i8 -75 ("Power (-100 to 100)\n0 = Stop/Brake\n-128 = Stop/Coast"), "Control Mode"="Power Only", "Controller Daisy Chain Position: 1 - 4"=u8 1, "Select Channel"="Motor 2") -> ()  [unwired: 3 in, 1 out]
          }
          frame True {
            n71 = call <vilib>:"TETRIX Motor Move_HT_myRIO.vi"("Power (-100 to 100)\n0 = Stop/Brake\n-128 = Stop/Coast"=100 ("Encoder Target: 360 = 1 motor shaft revolution"), "Control Mode"="Power Only", "Controller Daisy Chain Position: 1 - 4"=u8 1, "Select Channel"="Motor 2") -> ()  [unwired: 3 in, 1 out]
          }
        }
        n72 = call "Motor Control.vi"("error in (no error)"=w1135, "MotorSelect"=i16 2, "INSpeed"=w1126, "VISA Refnum in"=w1136) -> ("error out"=w1133:errorcluster, "VISA Refnum out"=w1134:refnum<visa-resource-name>)  [unwired: 6 in]
        n73 = global read "Global Var.vi" "ENA"() -> (w1152:bool)
        n74 = case shown="True" w1152 {
          frame False {
          }
          frame True {
            w1169 = FALSE ("LED camera")
            n75 = global write "Global Var.vi" "Motor_slide1"(FALSE ("LED camera")) -> ()
            n76 = global write "Global Var.vi" "Motor_rotate"(w1169) -> ()
            n77 = global write "Global Var.vi" "Motor_slide2"(w1169) -> ()
          }
        }
        n78 = global read "Global Var.vi" "Servo Camera"() -> (w1147:u8)
        n79 = call <vilib>:"TETRIX Servo Move_HT_myRIO.vi"("Servo Position (0 - 255)"=w1147, "Controller Daisy Chain Position (1 - 4)"=w1139, "Enable Sync: Fast | Medium | Slow | None"="None", "Select Servo"="Servo 6") -> ()  [unwired: 1 in, 1 out]
        n80 = global read "Global Var.vi" "INSpeed 3"() -> (w1127:dbl)
        n81 = global read "Global Var.vi" "Servo socket"() -> (w1146:u8)
        n82 = global read "Global Var.vi" "Servo_Arm_Kick_main"() -> (w1124:bool)
        n83 = case shown="True" w1124 {
          frame False {
            n84 = global write "Global Var.vi" "Servo Arm Kick"(u8 70 ("Servo Camera")) -> ()
          }
          frame True {
            n85 = global write "Global Var.vi" "Servo Arm Kick"(u8 170 ("Servo Camera")) -> ()
          }
        }
        n86 = call <vilib>:"TETRIX Servo Move_HT_myRIO.vi"("Servo Position (0 - 255)"=w1146, "Controller Daisy Chain Position (1 - 4)"=w1139, "Enable Sync: Fast | Medium | Slow | None"="None", "Select Servo"="Servo 5") -> ()  [unwired: 1 in, 1 out]
        n87 = global read "Global Var.vi" "Servo Gripper"() -> (w1145:u8)
        n88 = call "Motor Control.vi"("error in (no error)"=w1133, "MotorSelect"=i16 3, "INSpeed"=w1127, "VISA Refnum in"=w1134) -> ("error out"=w1131:errorcluster, "VISA Refnum out"=w1132:refnum<visa-resource-name>)  [unwired: 6 in]
        n89 = call <vilib>:"TETRIX Servo Move_HT_myRIO.vi"("Servo Position (0 - 255)"=w1145, "Controller Daisy Chain Position (1 - 4)"=w1139, "Enable Sync: Fast | Medium | Slow | None"="None", "Select Servo"="Servo 4") -> ()  [unwired: 1 in, 1 out]
        n90 = global read "Global Var.vi" "Servo Arm Kick"() -> (w1144:u8)
        n91 = global read "Global Var.vi" "Servo_Camera_main"() -> (w1123:bool)
        n92 = case shown="True" w1123 {
          frame False {
            n93 = global write "Global Var.vi" "Servo Camera"(u8 200 ("Servo Camera")) -> ()
          }
          frame True {
            n94 = global write "Global Var.vi" "Servo Camera"(u8 134 ("Servo Camera")) -> ()
          }
        }
        n95 = call <vilib>:"TETRIX Servo Move_HT_myRIO.vi"("Servo Position (0 - 255)"=w1144, "Controller Daisy Chain Position (1 - 4)"=w1139, "Enable Sync: Fast | Medium | Slow | None"="None", "Select Servo"="Servo 3") -> ()  [unwired: 1 in, 1 out]
        n96 = global read "Global Var.vi" "Servo Kick"() -> (w1143:u8)
        n97 = call <vilib>:"TETRIX Servo Move_HT_myRIO.vi"("Servo Position (0 - 255)"=w1143, "Controller Daisy Chain Position (1 - 4)"=w1139, "Enable Sync: Fast | Medium | Slow | None"="None", "Select Servo"="Servo 2") -> ()  [unwired: 1 in, 1 out]
        n98 = global read "Global Var.vi" "Servo Kick 2"() -> (w1140:u8)
        n99 = call <vilib>:"TETRIX Servo Move_HT_myRIO.vi"("Servo Position (0 - 255)"=w1140, "Controller Daisy Chain Position (1 - 4)"=w1139, "Enable Sync: Fast | Medium | Slow | None"="Fast", "Select Servo"="Servo 1") -> ()  [unwired: 1 in, 1 out]
      }
      n100 = while {
        shift-right: [w759] -> _
        shift-left: w69 -> [w799]
        shift-right: [w758] -> _
        shift-left: w69 -> [w800]
        shift-right: [w700] -> _
        shift-left: w69 -> [w801]
        shift-right: [w789] -> _
        shift-left: w70 -> [w790]
        shift-right: [w788] -> _
        shift-left: w70 -> [w791]
        shift-right: [w787] -> _
        shift-left: w70 -> [w792]
        stop <- w766 stop-if-true
        w794 = 100.0 ("y")
        w793 = 0.0 ("t")
        n101 = global read "Global Var.vi" "Mode PID"() -> (w751:bool)
        n102 = global read "Global Var.vi" "Encoder 1"() -> (w759:i32)
        n103 = global read "Global Var.vi" "Encoder 2"() -> (w758:i32)
        n104 = global read "Global Var.vi" "Encoder 3"() -> (w700:i32)
        n105 = global read "Global Var.vi" "Speed(rad/s) 1"() -> (w748:dbl)
        n106 = global read "Global Var.vi" "Speed(rad/s) 2"() -> (w747:dbl)
        n107 = global read "Global Var.vi" "Speed(rad/s) 3"() -> (w746:dbl)
        n108 = local read "OutX"() -> (w733:dbl)
        n109 = local read "OutY"() -> (w731:dbl)
        n110 = local read "OutTheta"() -> (w732:dbl)
        n111 = Wait (ms)(milliseconds to wait=u32 10) -> ()  [unwired: 1 out]
        n112 = global read "Global Var.vi" "Reset"() -> (w765:bool)
        n113 = case shown="False" w751 {
          tunnel: [w855 w898] -> w772
          tunnel: [w854 w897] -> w771
          tunnel: [w853 w893] -> w745
          frame False {
            w850 = 0.0 ("setpoint")
            # "30\n-30"
            n114 = global read "Global Var.vi" "Line Dis X"() -> (w842:bool)
            n115 = global read "Global Var.vi" "Line Dis"() -> (w856:bool)
            n116 = case shown="True" w842 {
              tunnel: [w857 w862] -> w852
              frame False {
                n117 = global read "Global Var.vi" "Set X"() -> (w857:dbl)
              }
              frame True {
                # "+-500"
                n118 = global read "Global Var.vi" "Speed Low"() -> (w858:bool)
                n119 = global read "Global Var.vi" "Line_X0"() -> (w859:dbl)
                n120 = global read "Global Var.vi" "X_Line"() -> (w860:dbl)
                n121 = case shown="True" w858 {
                  tunnel: [cluster{"output high":dbl, "output low":dbl} {"output high"=200.0, "output low"=-200.0} ("output range") cluster{"output high":dbl, "output low":dbl} {"output high"=50.0, "output low"=-50.0} ("output range")] -> w867
                  frame False {
                  }
                  frame True {
                  }
                }
                n122 = Bundle("Line_X0"=w859, "X_Line"=w860) -> (→"Chart Trackline":cluster{"Line_X0":dbl, "X_Line":dbl})  [unwired: 1 in]
                n123 = call-poly <vilib>:"PID.vi"("output range"=w867, "PID gains"="PID gains 4", "process variable"=w860, "setpoint"=w859) -> ("output"=w864:dbl)  [unwired: 6 in, 1 out]
                n124 = global read "Global Var.vi" "Status_line"() -> (w863:bool)
                n125 = Select(t=0.0, s=w863, f=w864) -> (s? t:f=w862:dbl)
              }
            }
            n126 = case shown="False" w856 {
              tunnel: [w870 w871] -> w855
              frame False {
                n127 = global read "Global Var.vi" "Set Y"() -> (w870:dbl)
              }
              frame True {
                n128 = global read "Global Var.vi" "Cross Line Position"() -> (w876:dbl)
                n129 = global read "Global Var.vi" "Cross set"() -> (w875:dbl)
                n130 = Bundle("Cross set"=w875, "Cross Line Position"=w876) -> (→"Chart Trackline 2":T13)  [unwired: 1 in]
                n131 = call-poly <vilib>:"PID.vi"("output range"=cluster{"output high":dbl, "output low":dbl} {"output high"=500.0, "output low"=-500.0}, "PID gains"="PID gains 5", "process variable"=w876, "setpoint"=w875) -> ("output"=w879:dbl)  [unwired: 6 in, 1 out]
                n132 = global read "Global Var.vi" "Status_Distance"() -> (w874:bool)
                n133 = Select(t=0.0, s=w874, f=w879) -> (s? t:f=w871:dbl)
              }
            }
            n134 = global read "Global Var.vi" "Angle_Line"() -> (w843:dbl)
            n135 = call-poly <vilib>:"PID.vi"("output range"=cluster{"output high":dbl, "output low":dbl} {"output high"=10.0, "output low"=-10.0}, "PID gains"="PID gains 6", "process variable"=w843, "setpoint"=w850) -> ("output"=w847:dbl)  [unwired: 6 in, 1 out]
            n136 = global read "Global Var.vi" "Theta_line"() -> (w846:bool)
            n137 = Bundle("setpoint"=w850, "Angle_Line"=w843) -> (→"Chart Trackline 3":cluster{"setpoint":dbl, "Angle_Line":dbl})  [unwired: 1 in]
            n138 = Select(t=0.0, s=w846, f=w847) -> (s? t:f=w845:dbl)
            n139 = Negate(x=w845) -> (-x=w853:dbl)
            n140 = Negate(x=w852) -> (-x=w854:dbl)
          }
          frame True {
            w880 = 100.0 ("y")
            w881 = 100.0 ("y")
            n141 = global read "Global Var.vi" "Y_set"() -> (w889:dbl)
            n142 = global read "Global Var.vi" "Y_en"() -> (w888:dbl)
            n143 = global read "Global Var.vi" "X_set"() -> (w885:dbl)
            n144 = global read "Global Var.vi" "X_en"() -> (w884:dbl)
            n145 = global read "Global Var.vi" "Theta_set"() -> (w891:dbl)
            n146 = global read "Global Var.vi" "Theta_en"() -> (w890:dbl)
            n147 = Multiply(x=w885, y=w881) -> (x*y=w883:dbl)
            n148 = Multiply(x=w884, y=w881) -> (x*y=w882:dbl)
            n149 = Multiply(x=w889, y=w880) -> (x*y=w886:dbl)
            n150 = Multiply(x=w888, y=w880) -> (x*y=w887:dbl)
            n151 = Bundle(w886, w887) -> (→"Chart Y":cluster{dbl, dbl})  [unwired: 1 in]
            n152 = call-poly <vilib>:"PID.vi"("output range"=cluster{"output high":dbl, "output low":dbl} {"output high"=3000.0, "output low"=-3000.0}, "PID gains"="PID gains", "process variable"=w882, "setpoint"=w883) -> ("output"=w904:dbl)  [unwired: 6 in, 1 out]
            n153 = Bundle(w883, w882) -> (→"Chart X":cluster{dbl, dbl})  [unwired: 1 in]
            n154 = Bundle("Theta_set"=w891, "Theta_en"=w890) -> (→"Chart Theta":cluster{"Theta_set":dbl, "Theta_en":dbl})  [unwired: 1 in]
            n155 = call-poly <vilib>:"PID.vi"("output range"=cluster{"output high":dbl, "output low":dbl} {"output high"=3000.0, "output low"=-3000.0}, "PID gains"="PID gains 2", "process variable"=w887, "setpoint"=w886) -> ("output"=w901:dbl)  [unwired: 6 in, 1 out]
            n156 = call-poly <vilib>:"PID.vi"("output range"=cluster{"output high":dbl, "output low":dbl} {"output high"=180.0, "output low"=-180.0}, "PID gains"="PID gains 3", "process variable"=w890, "setpoint"=w891) -> ("output"=w899:dbl)  [unwired: 6 in, 1 out]
            n157 = global read "Global Var.vi" "Status_theta"() -> (w894:bool)
            n158 = global read "Global Var.vi" "Status_x"() -> (w896:bool)
            n159 = global read "Global Var.vi" "Status_y"() -> (w895:bool)
            n160 = Select(t=0.0, s=w896, f=w904) -> (s? t:f=w897:dbl)
            n161 = Select(t=0.0, s=w895, f=w901) -> (s? t:f=w898:dbl)
            n162 = Select(t=0.0, s=w894, f=w899) -> (s? t:f=w893:dbl)
          }
        }
        "OutX" <- w771
        "OutY" <- w772
        "OutTheta" <- w745
        n163 = global read "Global Var.vi" "Reset"() -> (w764:bool)
        n164 = Subtract(x=w759, y=w799) -> (x-y=w725:i32)
        n165 = Subtract(x=w758, y=w800) -> (x-y=w723:i32)
        n166 = Subtract(x=w700, y=w801) -> (x-y=w722:i32)
        n167 = global read "Global Var.vi" "Theta_en"() -> (w712:dbl)
        n168 = Multiply(x=w732, y=50.0) -> (x*y=w774:dbl)
        n169 = call "Forward Kinematics.vi"("L(m)"=0.113, "r(m)"=0.019, "Phi3(rad/s)"=w746, "Phi2(rad/s)"=w747, "Phi1(rad/s)"=w748) -> ("Theta(deg/s)"=w713:dbl, "Y(m/s)"=w715:dbl, "X(m/s)"=w716:dbl)  [unwired: 4 in]
        n170 = Select(t=w793, s=w765, f=w791) -> (s? t:f=w796:dbl)
        n171 = Select(t=w793, s=w765, f=w792) -> (s? t:f=w797:dbl)
        n172 = Select(t=w793, s=w765, f=w790) -> (s? t:f=w795:dbl)
        n173 = xnode ("Encoder3")("Reset Counter"=w764) -> ("Counter Value"=w804:i32)  [unwired: 1 in, 3 out]
        n174 = xnode ("Encoder 2")("Reset Counter"=w764) -> ("Counter Value"=w803:i32)  [unwired: 1 in, 3 out]
        n175 = xnode ("Encoder1")("Reset Counter"=w764) -> ("Counter Value"=w802:i32)  [unwired: 1 in, 3 out]
        n176 = expression code="(x/180.0)*pi" "degrees to radians"(w712) -> (w711:dbl)
        n177 = Negate(x=w733) -> (-x=w779:dbl)
        n178 = Negate(x=w731) -> (-x=w778:dbl)
        n179 = Negate(x=w774) -> (-x=w773:dbl)
        n180 = Build Array(w716, w715) -> (w714:dbl[])
        n181 = Negate(x=w802) -> (-x=w760:i32)
        n182 = Negate(x=w803) -> (-x=w761:i32)
        n183 = Negate(x=w804) -> (-x=w762:i32)
        n184 = Build Array(w779, w778, w773) -> (w730:dbl[])
        n185 = global write "Global Var.vi" "Encoder 2"(w760) -> ()
        n186 = global write "Global Var.vi" "Encoder 3"(w761) -> ()
        n187 = global write "Global Var.vi" "Encoder 1"(w762) -> ()
        n188 = call "Pulse convert.vi"("PulseIN"=w725) -> ("Speed(rpm)"=w720:i16, "Speed(rad/s)"=w724:dbl)  [unwired: 9 in]
        n189 = call "Pulse convert.vi"("PulseIN"=w723) -> ("Speed(rpm)"=w719:i16, "Speed(rad/s)"=w721:dbl)  [unwired: 9 in]
        n190 = call "Pulse convert.vi"("PulseIN"=w722) -> ("Speed(rpm)"=w718:i16, "Speed(rad/s)"=w717:dbl)  [unwired: 9 in]
        n191 = call <vilib>:"Convert Global Velocity to Steering Frame.vi"("steering frame angle (rad)"=w711, "global velocity"=w730) -> ("steering frame velocity"=w729:dbl[])  [unwired: 9 in]
        n192 = call <vilib>:"Convert Steering Frame Velocity to Global.vi"("steering frame angle (rad)"=w711, "steering frame velocity"=w714) -> ("global velocity"=w710:dbl[])  [unwired: 9 in]
        n193 = Index Array(array=w710) -> (element #1=w709:dbl, element #2=w708:dbl)  [unwired: 2 in]
        n194 = Index Array(array=w729) -> (element #1=w780:dbl, element #2=w781:dbl, element #3=w782:dbl)  [unwired: 3 in]
        n195 = Add(x=w709, y=w795) -> (x+y=w789:dbl)
        n196 = Add(x=w708, y=w796) -> (x+y=w788:dbl)
        n197 = Add(x=w713, y=w797) -> (x+y=w787:dbl)
        n198 = global read "Global Var.vi" "ENA"() -> (w763:bool)
        n199 = call "Inverse Kinematics.vi"("r(m)"=0.019, "L(m)"=0.113 ("r(m)"), "Theta Set"=w782, "Y Set"=w781, "X Set"=w780) -> ("Out Motor 3"=w735:dbl, "Out Motor 2"=w736:dbl, "Out Motor 1"=w737:dbl)  [unwired: 4 in]
        n200 = global read "Global Var.vi" "Stop"() -> (w766:bool)
        n201 = Divide(x=w789, y=w794) -> (x/y=w784:dbl)
        n202 = Divide(x=w788, y=w794) -> (x/y=w783:dbl)
        n203 = Divide(x=w787, y=w794) -> (x/y=w727:dbl)
        n204 = global write "Global Var.vi" "Speed(rad/s) 1"(w724) -> ()
        n205 = global write "Global Var.vi" "Speed(rad/s) 2"(w721) -> ()
        n206 = global write "Global Var.vi" "Speed(rad/s) 3"(w717) -> ()
        n207 = global write "Global Var.vi" "Speed(rpm) 1"(w720) -> ()
        n208 = global write "Global Var.vi" "Speed(rpm) 2"(w719) -> ()
        n209 = global write "Global Var.vi" "Speed(rpm) 3"(w718) -> ()
        n210 = Negate(x=w784) -> (-x=w707:dbl)
        n211 = Negate(x=w783) -> (-x=w706:dbl)
        n212 = Multiply(x=w727, y=1.8000000000000003) -> (x*y=w728:dbl)
        n213 = xnode ("Digital output (1 sample)")("ENA (B/DIO0 (Pin 11))"=w763, "Qrcode (B/DIO2 (Pin 15))"=FALSE) -> ()  [unwired: 1 in, 1 out]
        n214 = global write "Global Var.vi" "INSpeed 1"(w737) -> ()
        n215 = global write "Global Var.vi" "INSpeed 2"(w736) -> ()
        n216 = global write "Global Var.vi" "INSpeed 3"(w735) -> ()
        n217 = global write "Global Var.vi" "Y_en"(w706) -> ()
        n218 = global write "Global Var.vi" "Theta_en"(w728) -> ()
        n219 = global write "Global Var.vi" "X_en"(w707) -> ()
        n220 = global read "Global Var.vi" "GoalT/F"() -> (w702:bool)
        n221 = case shown="True" w702 {
          frame False {
            n222 = global read "Global Var.vi" "Error robot 2"() -> (w812:dbl)
            n223 = global read "Global Var.vi" "Error robot 2"() -> (w811:dbl)
            n224 = global read "Global Var.vi" "Error theta 2"() -> (w808:dbl)
            n225 = global read "Global Var.vi" "Theta_set"() -> (w814:dbl)
            n226 = global read "Global Var.vi" "Theta_en"() -> (w813:dbl)
            n227 = global read "Global Var.vi" "Y_set"() -> (w810:dbl)
            n228 = global read "Global Var.vi" "Y_en"() -> (w809:dbl)
            n229 = global read "Global Var.vi" "X_set"() -> (w816:dbl)
            n230 = global read "Global Var.vi" "X_en"() -> (w815:dbl)
            n231 = Subtract(x=w816, y=w815) -> (x-y=w822:dbl)
            n232 = Subtract(x=w810, y=w809) -> (x-y=w820:dbl)
            n233 = Subtract(x=w814, y=w813) -> (x-y=w819:dbl)
            n234 = Absolute Value(x=w819) -> (abs(x)=w818:dbl)
            n235 = Absolute Value(x=w820) -> (abs(x)=w817:dbl)
            n236 = Absolute Value(x=w822) -> (abs(x)=w821:dbl)
            n237 = Less Or Equal?(x=w821, y=w812) -> (x <= y?=w807:bool)
            n238 = Less Or Equal?(x=w817, y=w811) -> (x <= y?=w805:bool)
            n239 = Less Or Equal?(x=w818, y=w808) -> (x <= y?=w806:bool)
            n240 = global write "Global Var.vi" "Status_x"(w807) -> ()
            n241 = global write "Global Var.vi" "Status_y"(w805) -> ()
            n242 = global write "Global Var.vi" "Status_theta"(w806) -> ()
          }
          frame True {
            n243 = global read "Global Var.vi" "Error robot"() -> (w830:dbl)
            n244 = global read "Global Var.vi" "Error robot"() -> (w829:dbl)
            n245 = global read "Global Var.vi" "Error theta"() -> (w826:dbl)
            n246 = global read "Global Var.vi" "Theta_set"() -> (w832:dbl)
            n247 = global read "Global Var.vi" "Theta_en"() -> (w831:dbl)
            n248 = global read "Global Var.vi" "Y_set"() -> (w828:dbl)
            n249 = global read "Global Var.vi" "Y_en"() -> (w827:dbl)
            n250 = global read "Global Var.vi" "X_set"() -> (w834:dbl)
            n251 = global read "Global Var.vi" "X_en"() -> (w833:dbl)
            n252 = Subtract(x=w834, y=w833) -> (x-y=w840:dbl)
            n253 = Subtract(x=w828, y=w827) -> (x-y=w838:dbl)
            n254 = Subtract(x=w832, y=w831) -> (x-y=w837:dbl)
            n255 = Absolute Value(x=w837) -> (abs(x)=w836:dbl)
            n256 = Absolute Value(x=w838) -> (abs(x)=w835:dbl)
            n257 = Absolute Value(x=w840) -> (abs(x)=w839:dbl)
            n258 = Less Or Equal?(x=w839, y=w830) -> (x <= y?=w825:bool)
            n259 = Less Or Equal?(x=w835, y=w829) -> (x <= y?=w823:bool)
            n260 = Less Or Equal?(x=w836, y=w826) -> (x <= y?=w824:bool)
            n261 = global write "Global Var.vi" "Status_x"(w825) -> ()
            n262 = global write "Global Var.vi" "Status_y"(w823) -> ()
            n263 = global write "Global Var.vi" "Status_theta"(w824) -> ()
          }
        }
        n264 = global read "Global Var.vi" "Cross Line Position"() -> (w753:dbl)
        n265 = global read "Global Var.vi" "Error Angle Line"() -> (w734:dbl)
        n266 = global read "Global Var.vi" "Error Distance"() -> (w752:dbl)
        n267 = global read "Global Var.vi" "Angle_Line"() -> (w741:dbl)
        n268 = global read "Global Var.vi" "Cross set"() -> (w754:dbl)
        n269 = global read "Global Var.vi" "Error line"() -> (w755:dbl)
        n270 = global read "Global Var.vi" "Line_X0"() -> (w757:dbl)
        n271 = global read "Global Var.vi" "X_Line"() -> (w756:dbl)
        n272 = case shown="True" "Set 0" {
          frame False {
          }
          frame True {
            w841 = 0.0 ("Theta_set")
            n273 = global write "Global Var.vi" "Theta_set"(w841) -> ()
            n274 = global write "Global Var.vi" "X_set"(w841) -> ()
            n275 = global write "Global Var.vi" "Y_set"(w841) -> ()
          }
        }
        n276 = xnode ("Digital input (1 sample)")() -> ("Start_SW (A/DIO7 (Pin 25))"=w704:bool, "Limit_Gripper (B/DIO1 (Pin 13))"=w703:bool)  [unwired: 1 in, 1 out]
        n277 = Subtract(x=w757, y=w756) -> (x-y=w769:dbl)
        n278 = Subtract(x=w754, y=w753) -> (x-y=w768:dbl)
        n279 = Subtract(x=0.0, y=w741) -> (x-y=w743:dbl)
        n280 = Not(x=w704) -> (.not. x?=w744:bool)
        n281 = Not(x=w703) -> (.not. x?=w738:bool)
        n282 = Absolute Value(x=w769) -> (abs(x)=w770:dbl)
        n283 = Absolute Value(x=w768) -> (abs(x)=w767:dbl)
        n284 = Absolute Value(x=w743) -> (abs(x)=w742:dbl)
        n285 = Less Or Equal?(x=w770, y=w755) -> (x <= y?=w749:bool)
        n286 = global write "Global Var.vi" "Limit Gripper"(w738) -> ()
        n287 = Less Or Equal?(x=w767, y=w752) -> (x <= y?=w750:bool)
        n288 = Less Or Equal?(x=w742, y=w734) -> (x <= y?=w740:bool)
        n289 = global write "Global Var.vi" "Start_SW"(w744) -> ()
        n290 = global write "Global Var.vi" "Theta_line"(w740) -> ()
        n291 = global write "Global Var.vi" "Status_line"(w749) -> ()
        n292 = global write "Global Var.vi" "Status_Distance"(w750) -> ()
      }
      n293 = while {
        shift-right: [w193] -> _
        shift-left: w68 -> [w194]
        stop <- w195 stop-if-true
        n294 = global read "Global Var.vi" "Stop"() -> (w195:bool)
        n295 = case shown="103" w194 {
          tunnel: [0 w252 3 4 w268 27 27 8 w298 w343 8 27 13 27 15 16 17 w381 103 w425 27 w435 w440 w445 w485 103 1 111 107 107 107 w535 103 103 103 112 1 100 w566 103 w600 103 w636 112 w669 210] -> w193
          frame 0 {
            w200 = 0.0 ("X_set")
            n296 = global write "Global Var.vi" "Servo Gripper"(u8 110 ("Servo Camera")) -> ()
            n297 = global write "Global Var.vi" "Servo Kick"(u8 0 ("Servo Camera")) -> ()
            n298 = global write "Global Var.vi" "Servo Arm Kick"(u8 30 ("Servo Camera")) -> ()
            n299 = global write "Global Var.vi" "Servo socket"(u8 100 ("Servo Camera")) -> ()
            n300 = global write "Global Var.vi" "Mode PID"(TRUE ("Mode PID")) -> ()
            n301 = global write "Global Var.vi" "Line Dis"(FALSE ("Mode PID")) -> ()
            n302 = global write "Global Var.vi" "Theta_set"(w200) -> ()
            n303 = global write "Global Var.vi" "X_set"(w200) -> ()
            n304 = global write "Global Var.vi" "Y_set"(w200) -> ()
            n305 = global write "Global Var.vi" "Reset"(TRUE ("ENA")) -> ()
            n306 = global write "Global Var.vi" "Vision Mode"(u8 6 ("Servo Camera")) -> ()
            n307 = disable-structure shown="Disabled" {
              frame Disabled {
                w218 = i16 0 ("INSpeed 1")
                n308 = global read "Global Var.vi" "Start_SW"() -> (w215:bool)
                n309 = global write "Global Var.vi" "Motor_slide1"(FALSE ("ENA")) -> ()
                n310 = global write "Global Var.vi" "Motor_rotate"(FALSE ("ENA")) -> ()
                n311 = global write "Global Var.vi" "Motor_slide2"(FALSE ("LED camera")) -> ()
                n312 = global write "Global Var.vi" "ENA"(FALSE ("ENA")) -> ()
                n313 = global write "Global Var.vi" "ENA"(TRUE ("ENA")) -> ()
                n314 = global write "Global Var.vi" "Stop"(w215) -> ()
                n315 = global write "Global Var.vi" "Set Y"("Set Y") -> ()
                n316 = global write "Global Var.vi" "INSpeed 1"(w218) -> ()
                n317 = global write "Global Var.vi" "INSpeed 2"(w218) -> ()
                n318 = global write "Global Var.vi" "INSpeed 3"(w218) -> ()
                n319 = global write "Global Var.vi" "Reset"(FALSE ("ENA")) -> ()
              }
              frame Enabled {
              }
            }
            n320 = global write "Global Var.vi" "Servo_Camera_main"(TRUE ("Mode PID")) -> ()
            n321 = global write "Global Var.vi" "LED camera"(TRUE ("Mode PID")) -> ()
            n322 = global write "Global Var.vi" "QRCodeTick"("QRCodeTick") -> ()
          }
          frame 1, Default {
            w245 = 0.0 ("X_set")
            # "รอกดสวิตซ์เริ่ม"
            n323 = global write "Global Var.vi" "Servo Kick 2"(u8 255 ("Servo Camera")) -> ()
            n324 = global write "Global Var.vi" "Servo Gripper"(u8 110 ("Servo Camera")) -> ()
            n325 = global write "Global Var.vi" "Servo Kick"(u8 200 ("Servo Camera")) -> ()
            n326 = global write "Global Var.vi" "Theta_set"(w245) -> ()
            n327 = global write "Global Var.vi" "Servo socket"(u8 150 ("Servo Camera")) -> ()
            n328 = global write "Global Var.vi" "Speed Low"(FALSE ("Mode PID")) -> ()
            n329 = global write "Global Var.vi" "Mode PID"(TRUE ("Mode PID")) -> ()
            n330 = global write "Global Var.vi" "ENA"(TRUE ("ENA")) -> ()
            n331 = global write "Global Var.vi" "X_set"(w245) -> ()
            n332 = global write "Global Var.vi" "Y_set"(w245) -> ()
            n333 = global write "Global Var.vi" "Vision Mode"(i16 0 ("Vision Mode")) -> ()
            n334 = global write "Global Var.vi" "Reset"(TRUE ("ENA")) -> ()
            n335 = global write "Global Var.vi" "QRCodeTick"(FALSE ("Mode PID")) -> ()
            n336 = global write "Global Var.vi" "Motor_slide1"(FALSE ("Mode PID")) -> ()
            n337 = global write "Global Var.vi" "Motor_rotate"(FALSE ("ENA")) -> ()
            n338 = global write "Global Var.vi" "LED camera"(TRUE ("LED camera")) -> ()
            n339 = global write "Global Var.vi" "Motor_slide2"(FALSE ("ENA")) -> ()
            n340 = global write "Global Var.vi" "Stock"(i16 0 ("Stock")) -> ()
            n341 = global write "Global Var.vi" "BlueBox"(i16 7 ("BlueBox")) -> ()
            n342 = global write "Global Var.vi" "BlueBox (blue)"(i16 2 ("BlueBox")) -> ()
            n343 = global write "Global Var.vi" "BlueBox (red)"(i16 4 ("BlueBox")) -> ()
            n344 = global write "Global Var.vi" "BlueBox (yellow)"(i16 1 ("BlueBox")) -> ()
            n345 = local write "Reset"(FALSE ("Reset")) -> ()
            n346 = global write "Global Var.vi" "Line Dis X"(TRUE ("Mode PID")) -> ()
            n347 = global write "Global Var.vi" "Color Box"(u32 6618880 ("Color Box")) -> ()
            n348 = global write "Global Var.vi" "RedBox"(i16 7 ("RedBox")) -> ()
            n349 = global write "Global Var.vi" "RedBox (blue)"(i16 4 ("BlueBox")) -> ()
            n350 = global write "Global Var.vi" "RedBox (red)"(i16 2 ("BlueBox")) -> ()
            n351 = global write "Global Var.vi" "RedBox (yellow)"(i16 1 ("BlueBox")) -> ()
            n352 = global write "Global Var.vi" "Status"("รอกดสวิตซ์เริ่ม" ("Status")) -> ()
            n353 = global write "Global Var.vi" "Servo_Arm_Kick_main"(FALSE ("Mode PID")) -> ()
            n354 = global write "Global Var.vi" "Servo_Camera_main"(FALSE ("Mode PID")) -> ()
            n355 = disable-structure shown="Disabled" {
              frame Disabled {
                n356 = global write "Global Var.vi" "Servo Camera"(u8 200 ("Servo Camera")) -> ()
                n357 = global write "Global Var.vi" "Servo Arm Kick"(u8 70 ("Servo Camera")) -> ()
              }
              frame Enabled {
              }
            }
            n358 = global read "Global Var.vi" "Start_SW"() -> (w223:bool)
            n359 = case shown="True" w223 {
              frame False {
              }
              frame True {
                n360 = local read "time"() -> (w255:u32)
                n361 = local write "lasttime"(w255) -> ()
              }
            }
            n362 = Select(t=2, s=w223, f=1) -> (s? t:f=w252:i32)
          }
          frame 2 {
            # "วื่งจากจุด Start ไปที่โซน แดง"
            n363 = call "Step1to2.vi"() -> ()  [unwired: 12 in]
            n364 = global write "Global Var.vi" "Color Box"(u32 16711680 ("Color Box")) -> ()
          }
          frame 3 {
            # "4"
            # "ทำการหยิบลูกแรก"
            n365 = call "StepPick.vi"() -> ()  [unwired: 12 in]
            n366 = global read "Global Var.vi" "RedBox"() -> (w259:i16)
            n367 = global write "Global Var.vi" "BlueBox"(i16 7 ("BlueBox")) -> ()
            n368 = Decrement(x=w259) -> (x-1=w260:i16)
            n369 = global write "Global Var.vi" "Color Box"(u32 16711680 ("Color Box")) -> ()
            n370 = global write "Global Var.vi" "RedBox"(w260) -> ()
          }
          frame 4 {
            # "เช็คสีลูก"
            n371 = global read "Global Var.vi" "Color"() -> (w267:string)
            n372 = global write "Global Var.vi" "Color Box"(u32 16711680 ("Color Box")) -> ()
            n373 = global write "Global Var.vi" "Vision Mode"(i16 2 ("Vision Mode")) -> ()
            n374 = global write "Global Var.vi" "Status"("Color Detection" ("Status")) -> ()
            n375 = global write "Global Var.vi" "LED camera"(TRUE ("LED camera")) -> ()
            n376 = case shown="\"No Color\", Default" w267 {
              tunnel: [5 w273 4 7] -> w268
              frame "Red" {
              }
              frame "Blue" {
                n377 = global read "Global Var.vi" "Stock"() -> (w272:i16)
                n378 = Equal?(x=w272, y=i16 2) -> (x = y?=w270:bool)
                n379 = case shown="False" w270 {
                  tunnel: [6 w280] -> w273
                  frame False {
                    n380 = global read "Global Var.vi" "Stock"() -> (w276:i16)
                    n381 = Increment(x=w276) -> (x+1=w275:i16)
                    n382 = global write "Global Var.vi" "Stock"(w275) -> ()
                  }
                  frame True {
                    n383 = global read "Global Var.vi" "RedBox"() -> (w279:i16)
                    n384 = Equal?(x=w279, y=i16 0) -> (x = y?=w277:bool)
                    n385 = case shown="True" w277 {
                      tunnel: [5 6] -> w280
                      frame False {
                      }
                      frame True {
                        n386 = global read "Global Var.vi" "Stock"() -> (w282:i16)
                        n387 = Increment(x=w282) -> (x+1=w283:i16)
                        n388 = global write "Global Var.vi" "Stock"(w283) -> ()
                      }
                    }
                  }
                }
              }
              frame "No Color", Default {
              }
              frame "Yellow" {
              }
            }
          }
          frame 5 {
            # "สีแดง"
            n389 = call "Red Place.vi"() -> ()  [unwired: 12 in]
            n390 = global write "Global Var.vi" "Color Box"(u32 16711680 ("Color Box")) -> ()
          }
          frame 6 {
            # "สีน้ำเงิน"
            n391 = call "Blue Stock.vi"() -> ()  [unwired: 12 in]
            n392 = global write "Global Var.vi" "Color Box"(u32 16711680 ("Color Box")) -> ()
          }
          frame 7 {
            # "สีเหลือง"
            n393 = call "Red to Yellow1.vi"() -> ()  [unwired: 12 in]
            n394 = global write "Global Var.vi" "Yellow No"("1" ("Yellow No")) -> ()
            n395 = global write "Global Var.vi" "Color Box"(u32 16776722 ("Color Box")) -> ()
            n396 = global write "Global Var.vi" "Qrcode"(i16 4 ("Qrcode")) -> ()
          }
          frame 8 {
            w301 = i16 0 ("INSpeed 1")
            w302 = 0.0 ("X_set")
            # "เช็ค QRcode"
            n397 = global write "Global Var.vi" "Servo Kick"(u8 200 ("Servo Camera")) -> ()
            n398 = global write "Global Var.vi" "Servo Gripper"(u8 110 ("Servo Camera")) -> ()
            n399 = global write "Global Var.vi" "Servo socket"(u8 150 ("Servo Camera")) -> ()
            n400 = global write "Global Var.vi" "INSpeed 1"(w301) -> ()
            n401 = global write "Global Var.vi" "INSpeed 2"(w301) -> ()
            n402 = global write "Global Var.vi" "INSpeed 3"(w301) -> ()
            n403 = global read "Global Var.vi" "Qrcode"() -> (w299:i16)
            n404 = global write "Global Var.vi" "Status"("QRcode Detection" ("Status")) -> ()
            n405 = global read "Global Var.vi" "Qrcode"() -> (w297:i16)
            n406 = global write "Global Var.vi" "Theta_set"(w302) -> ()
            n407 = global write "Global Var.vi" "X_set"(w302) -> ()
            n408 = global write "Global Var.vi" "Y_set"(w302) -> ()
            n409 = global write "Global Var.vi" "Color Box"(u32 16776722 ("Color Box")) -> ()
            n410 = Equal?(x=w297, y=i16 4) -> (x = y?=w300:bool)
            n411 = case shown="3" w299 {
              tunnel: [w316 w324 8 w333] -> w298
              frame 3 {
                (unwired) 10
                n412 = flat-sequence {
                  tunnel: [10] -> w316
                  frame #0 {
                    n413 = global read "Global Var.vi" "Place_pos"() -> (w317:dbl)
                    n414 = Increment(x=w317) -> (x+1=w318:dbl)
                    n415 = global write "Global Var.vi" "Place_pos"(w318) -> ()
                  }
                  frame #1 {
                    n416 = global read "Global Var.vi" "Place_pos"() -> (w319:dbl)
                    n417 = case shown="1, Default" w319 {
                      frame 2 {
                        n418 = global write "Global Var.vi" "Place 2"(3.0 ("Place 1")) -> ()
                      }
                      frame 3 {
                        n419 = global write "Global Var.vi" "Place 3"(3.0 ("Place 1")) -> ()
                      }
                      frame 1, Default {
                        n420 = global write "Global Var.vi" "Place 1"(3.0 ("Place 1")) -> ()
                      }
                    }
                  }
                  frame #2 {
                  }
                }
              }
              frame 2 {
                n421 = flat-sequence {
                  tunnel: [10] -> w324
                  frame #0 {
                    n422 = global read "Global Var.vi" "Place_pos"() -> (w325:dbl)
                    n423 = Increment(x=w325) -> (x+1=w326:dbl)
                    n424 = global write "Global Var.vi" "Place_pos"(w326) -> ()
                  }
                  frame #1 {
                    n425 = global read "Global Var.vi" "Place_pos"() -> (w327:dbl)
                    n426 = case shown="1, Default" w327 {
                      frame 2 {
                        n427 = global write "Global Var.vi" "Place 2"(2.0 ("Place 1")) -> ()
                      }
                      frame 3 {
                        n428 = global write "Global Var.vi" "Place 3"(2.0 ("Place 1")) -> ()
                      }
                      frame 1, Default {
                        n429 = global write "Global Var.vi" "Place 1"(2.0 ("Place 1")) -> ()
                      }
                    }
                  }
                  frame #2 {
                  }
                }
              }
              frame 4, Default {
              }
              frame 1 {
                n430 = flat-sequence {
                  tunnel: [9] -> w333
                  frame #0 {
                    n431 = global read "Global Var.vi" "Place_pos"() -> (w334:dbl)
                    n432 = Increment(x=w334) -> (x+1=w335:dbl)
                    n433 = global write "Global Var.vi" "Place_pos"(w335) -> ()
                  }
                  frame #1 {
                    n434 = global read "Global Var.vi" "Place_pos"() -> (w336:dbl)
                    n435 = case shown="1, Default" w336 {
                      frame 2 {
                        n436 = global write "Global Var.vi" "Place 2"(1.0 ("Place 1")) -> ()
                      }
                      frame 3 {
                        n437 = global write "Global Var.vi" "Place 3"(1.0 ("Place 1")) -> ()
                      }
                      frame 1, Default {
                        n438 = global write "Global Var.vi" "Place 1"(1.0 ("Place 1")) -> ()
                      }
                    }
                  }
                  frame #2 {
                  }
                }
              }
            }
            n439 = case shown="True" w300 {
              frame False {
                n440 = global write "Global Var.vi" "QRCodeTick"(FALSE ("ENA")) -> ()
              }
              frame True {
                n441 = global write "Global Var.vi" "QRCodeTick"(TRUE ("ENA")) -> ()
              }
            }
            n442 = global write "Global Var.vi" "Mode PID"(TRUE ("Mode PID")) -> ()
            n443 = global write "Global Var.vi" "ENA"(TRUE ("ENA")) -> ()
            n444 = global write "Global Var.vi" "Reset"(TRUE ("ENA")) -> ()
            n445 = global write "Global Var.vi" "Line Dis"(FALSE ("Mode PID")) -> ()
            n446 = global write "Global Var.vi" "Vision Mode"(i16 0 ("Vision Mode")) -> ()
            n447 = global write "Global Var.vi" "Motor_slide1"(FALSE ("ENA")) -> ()
            n448 = global write "Global Var.vi" "Motor_rotate"(FALSE ("ENA")) -> ()
            n449 = global write "Global Var.vi" "LED camera"(FALSE ("Mode PID")) -> ()
            n450 = global write "Global Var.vi" "Motor_slide2"(FALSE ("LED camera")) -> ()
          }
          frame 9 {
            # "วางสีเหลือง"
            n451 = call "Yellow Place.vi"() -> ()  [unwired: 12 in]
            n452 = global write "Global Var.vi" "QRCodeTick"(FALSE ("Mode PID")) -> ()
            n453 = global write "Global Var.vi" "Qrcode"(i16 4 ("Qrcode")) -> ()
            n454 = global write "Global Var.vi" "Yellow No"("1" ("Yellow No")) -> ()
            n455 = global read "Global Var.vi" "Place_pos"() -> (w344:dbl)
            n456 = global write "Global Var.vi" "Color Box"(u32 16776722 ("Color Box")) -> ()
            n457 = case shown="2" w344 {
              tunnel: [13 26 28] -> w343
              frame 2 {
              }
              frame 3 {
              }
              frame 1, Default {
              }
            }
          }
          frame 10 {
            # "ย้ายตำแหน่ง Qrcode"
            n458 = global write "Global Var.vi" "Yellow No"("2" ("Yellow No")) -> ()
            n459 = global write "Global Var.vi" "Qrcode"(i16 4 ("Qrcode")) -> ()
            n460 = global write "Global Var.vi" "QRCodeTick"(FALSE ("Mode PID")) -> ()
            n461 = call "Yellow 1 to 2.vi"() -> ()  [unwired: 12 in]
            n462 = global write "Global Var.vi" "Color Box"(u32 16776722 ("Color Box")) -> ()
          }
          frame 11 {
            n463 = call "Yellow to Red 1.vi"() -> ()  [unwired: 12 in]
            n464 = global write "Global Var.vi" "Status"("กลับสีแดง" ("Status")) -> ()
            n465 = global write "Global Var.vi" "Color Box"(u32 16711680 ("Color Box")) -> ()
          }
          frame 12 {
            # "วางสีเหลือง2"
            n466 = call "Yellow Place.vi"() -> ()  [unwired: 12 in]
            n467 = global write "Global Var.vi" "QRCodeTick"(FALSE ("Mode PID")) -> ()
            n468 = global write "Global Var.vi" "Qrcode"(i16 4 ("Qrcode")) -> ()
            n469 = global write "Global Var.vi" "Yellow No"("2" ("Yellow No")) -> ()
            n470 = global write "Global Var.vi" "Color Box"(u32 16776722 ("Color Box")) -> ()
          }
          frame 13 {
            n471 = call "Yellow to Red 2.vi"() -> ()  [unwired: 12 in]
            n472 = global write "Global Var.vi" "Color Box"(u32 16711680 ("Color Box")) -> ()
            n473 = global write "Global Var.vi" "Status"("กลับสีแดง" ("Status")) -> ()
          }
          frame 14 {
            n474 = call "ZoneRed to ZoneBlue.vi"() -> ()  [unwired: 12 in]
            n475 = global write "Global Var.vi" "Stock"(i16 0 ("Stock")) -> ()
          }
          frame 15 {
            n476 = call "ZoneBlue rotatePlace.vi"() -> ()  [unwired: 12 in]
            n477 = global write "Global Var.vi" "Status"("ปล่อยลูก Blue" ("Status")) -> ()
          }
          frame 16 {
            # "17"
            # "หยิบลูกสีน้ำเงิน"
            n478 = global read "Global Var.vi" "BlueBox"() -> (w375:i16)
            n479 = call "StepPick_zone_Blue.vi"() -> ()  [unwired: 12 in]
            n480 = Decrement(x=w375) -> (x-1=w374:i16)
            n481 = global write "Global Var.vi" "BlueBox"(w374) -> ()
            n482 = global write "Global Var.vi" "Status"("หยิบลูก Blue" ("Status")) -> ()
            n483 = global write "Global Var.vi" "Color Box"(u32 2766079 ("Color Box")) -> ()
            n484 = disable-structure shown="Disabled" {
              frame Disabled {
                n485 = global write "Global Var.vi" "Place 1"(2.0 ("Place 3")) -> ()
                n486 = global write "Global Var.vi" "Place 2"(1.0 ("Place 3")) -> ()
                n487 = global write "Global Var.vi" "Place 3"(3.0 ("Place 3")) -> ()
              }
              frame Enabled {
              }
            }
          }
          frame 17 {
            # "เช็คสีลูก"
            n488 = global write "Global Var.vi" "Color Box"(u32 7821823 ("Color Box")) -> ()
            n489 = global write "Global Var.vi" "Vision Mode"(i16 2 ("Vision Mode")) -> ()
            n490 = global read "Global Var.vi" "Color"() -> (w386:string)
            n491 = global write "Global Var.vi" "Status"("Color Detection" ("Status")) -> ()
            n492 = global write "Global Var.vi" "Status"("เช็คสี Blue" ("Status")) -> ()
            n493 = case shown="\"Red\"" w386 {
              tunnel: [w387 18 17 w405] -> w381
              frame "Red" {
                # "18"
                n494 = global read "Global Var.vi" "Stock"() -> (w390:i16)
                n495 = Equal?(x=w390, y=i16 2) -> (x = y?=w388:bool)
                n496 = case shown="True" w388 {
                  tunnel: [19 w397] -> w387
                  frame False {
                    n497 = global read "Global Var.vi" "Stock"() -> (w393:i16)
                    n498 = Increment(x=w393) -> (x+1=w392:i16)
                    n499 = global write "Global Var.vi" "Stock"(w392) -> ()
                  }
                  frame True {
                    n500 = global read "Global Var.vi" "BlueBox (yellow)"() -> (w396:i16)
                    n501 = Equal?(x=w396, y=i16 0) -> (x = y?=w394:bool)
                    n502 = case shown="True" w394 {
                      tunnel: [18 19] -> w397
                      frame False {
                      }
                      frame True {
                        n503 = global read "Global Var.vi" "Stock"() -> (w399:i16)
                        n504 = Increment(x=w399) -> (x+1=w400:i16)
                        n505 = global write "Global Var.vi" "Stock"(w400) -> ()
                      }
                    }
                  }
                }
              }
              frame "Blue" {
              }
              frame "No Color", Default {
              }
              frame "Yellow" {
                n506 = global read "Global Var.vi" "Place 1"() -> (w420:dbl)
                n507 = global read "Global Var.vi" "Place 2"() -> (w418:dbl)
                n508 = global read "Global Var.vi" "Place 3"() -> (w416:dbl)
                n509 = Equal?(x=w420, y=2.0) -> (x = y?=w414:bool)
                n510 = Equal?(x=w418, y=2.0) -> (x = y?=w410:bool)
                n511 = Equal?(x=w416, y=2.0) -> (x = y?=w407:bool)
                n512 = global write "Global Var.vi" "BlueBox (yellow)"(i16 0 ("BlueBox (yellow)")) -> ()
                n513 = Select(t=106, s=w407, f=17) -> (s? t:f=w408:i32)
                n514 = Select(t=105, s=w410, f=w408) -> (s? t:f=w411:i32)
                n515 = Select(t=104, s=w414, f=w411) -> (s? t:f=w405:i32)
              }
            }
            n516 = global write "Global Var.vi" "LED camera"(TRUE ("LED camera")) -> ()
          }
          frame 18 {
            n517 = global write "Global Var.vi" "Status"("วาง Blue" ("Status")) -> ()
            n518 = call "Blue Place.vi"() -> ()  [unwired: 12 in]
            n519 = global write "Global Var.vi" "Color Box"(u32 2766079 ("Color Box")) -> ()
          }
          frame 19 {
            # "สีน้ำเงิน"
            n520 = global write "Global Var.vi" "Status"("เก็บRed zone Blue" ("Status")) -> ()
            n521 = call "Red Stock.vi"() -> ()  [unwired: 12 in]
            n522 = global write "Global Var.vi" "Color Box"(u32 7821823 ("Color Box")) -> ()
            n523 = global read "Global Var.vi" "Stock"() -> (w429:i16)
            n524 = Less?(x=w429, y=i16 2) -> (x < y?=w427:bool)
            n525 = Select(t=16, s=w427, f=103) -> (s? t:f=w425:i32)
          }
          frame 26 {
            n526 = call "Yellow to Red 3.vi"() -> ()  [unwired: 12 in]
            n527 = global write "Global Var.vi" "Color Box"(u32 16711680 ("Color Box")) -> ()
            n528 = global write "Global Var.vi" "Status"("กลับสีแดง" ("Status")) -> ()
          }
          frame 27 {
            n529 = global read "Global Var.vi" "RedBox"() -> (w439:i16)
            n530 = Greater Than 0?(x=w439) -> (x > 0?=w438:bool)
            n531 = Select(t=3, s=w438, f=14) -> (s? t:f=w435:i32)
          }
          frame 28 {
            n532 = flat-sequence {
              tunnel: [29] -> w440
              frame #0 {
                n533 = call "Yellow 1 to 2_spacial.vi"() -> ()  [unwired: 12 in]
              }
              frame #1 {
              }
            }
          }
          frame 29 {
            w448 = i16 0 ("INSpeed 1")
            w449 = 0.0 ("X_set")
            # "เช็ค QRcode"
            n534 = global write "Global Var.vi" "INSpeed 1"(w448) -> ()
            n535 = global write "Global Var.vi" "Servo Gripper"(u8 110 ("Servo Camera")) -> ()
            n536 = global write "Global Var.vi" "Servo Kick"(u8 200 ("Servo Camera")) -> ()
            n537 = global write "Global Var.vi" "Servo socket"(u8 150 ("Servo Camera")) -> ()
            n538 = global write "Global Var.vi" "INSpeed 2"(w448) -> ()
            n539 = global write "Global Var.vi" "INSpeed 3"(w448) -> ()
            n540 = global read "Global Var.vi" "Qrcode"() -> (w446:i16)
            n541 = global write "Global Var.vi" "Status"("QR 2 พิเศษ" ("Status")) -> ()
            n542 = global read "Global Var.vi" "Qrcode"() -> (w444:i16)
            n543 = global write "Global Var.vi" "Theta_set"(w449) -> ()
            n544 = global write "Global Var.vi" "X_set"(w449) -> ()
            n545 = global write "Global Var.vi" "Y_set"(w449) -> ()
            n546 = global write "Global Var.vi" "Color Box"(u32 16776722 ("Color Box")) -> ()
            n547 = Equal?(x=w444, y=i16 4) -> (x = y?=w447:bool)
            n548 = case shown="2" w446 {
              tunnel: [w463 w472 29 29] -> w445
              frame 3 {
                (unwired) 10
                n549 = flat-sequence {
                  tunnel: [13] -> w463
                  frame #0 {
                    n550 = global read "Global Var.vi" "Place_pos"() -> (w464:dbl)
                    n551 = Increment(x=w464) -> (x+1=w465:dbl)
                    n552 = global write "Global Var.vi" "Place_pos"(w465) -> ()
                  }
                  frame #1 {
                    n553 = global read "Global Var.vi" "Place_pos"() -> (w466:dbl)
                    n554 = case shown="3" w466 {
                      frame 2 {
                        n555 = global write "Global Var.vi" "Place 3"(2.0 ("Place 1")) -> ()
                        n556 = global write "Global Var.vi" "Place 2"(3.0 ("Place 1")) -> ()
                      }
                      frame 3 {
                        n557 = global write "Global Var.vi" "Place 3"(3.0 ("Place 1")) -> ()
                      }
                      frame 1, Default {
                        n558 = global write "Global Var.vi" "Place 1"(3.0 ("Place 1")) -> ()
                      }
                    }
                  }
                  frame #2 {
                  }
                }
              }
              frame 2 {
                n559 = flat-sequence {
                  tunnel: [13] -> w472
                  frame #0 {
                    n560 = global read "Global Var.vi" "Place_pos"() -> (w473:dbl)
                    n561 = Increment(x=w473) -> (x+1=w474:dbl)
                    n562 = global write "Global Var.vi" "Place_pos"(w474) -> ()
                  }
                  frame #1 {
                    n563 = global read "Global Var.vi" "Place_pos"() -> (w475:dbl)
                    n564 = case shown="2" w475 {
                      frame 2 {
                        n565 = global write "Global Var.vi" "Place 2"(2.0 ("Place 1")) -> ()
                        n566 = global write "Global Var.vi" "Place 3"(3.0 ("Place 1")) -> ()
                      }
                      frame 3 {
                        n567 = global write "Global Var.vi" "Place 3"(2.0 ("Place 1")) -> ()
                      }
                      frame 1, Default {
                        n568 = global write "Global Var.vi" "Place 1"(2.0 ("Place 1")) -> ()
                      }
                    }
                  }
                  frame #2 {
                  }
                }
              }
              frame 4, Default {
              }
              frame 1 {
              }
            }
            n569 = case shown="True" w447 {
              frame False {
                n570 = global write "Global Var.vi" "QRCodeTick"(FALSE ("ENA")) -> ()
              }
              frame True {
                n571 = global write "Global Var.vi" "QRCodeTick"(TRUE ("ENA")) -> ()
              }
            }
            n572 = global write "Global Var.vi" "Mode PID"(TRUE ("Mode PID")) -> ()
            n573 = global write "Global Var.vi" "ENA"(TRUE ("ENA")) -> ()
            n574 = global write "Global Var.vi" "Reset"(TRUE ("ENA")) -> ()
            n575 = global write "Global Var.vi" "Line Dis"(FALSE ("Mode PID")) -> ()
            n576 = global write "Global Var.vi" "Vision Mode"(i16 0 ("Vision Mode")) -> ()
            n577 = global write "Global Var.vi" "Motor_slide1"(FALSE ("ENA")) -> ()
            n578 = global write "Global Var.vi" "Motor_rotate"(FALSE ("ENA")) -> ()
            n579 = global write "Global Var.vi" "LED camera"(FALSE ("Mode PID")) -> ()
            n580 = global write "Global Var.vi" "Motor_slide2"(FALSE ("LED camera")) -> ()
          }
          frame 100 {
            w510 = 0.0 ("X_set")
            # "มุมตั้งตรง"
            # "มุม Track line"
            n581 = global write "Global Var.vi" "Servo Gripper"(u8 110 ("Servo Camera")) -> ()
            n582 = global write "Global Var.vi" "Servo Kick"(u8 200 ("Servo Camera")) -> ()
            n583 = global write "Global Var.vi" "Servo socket"(u8 150 ("Servo Camera")) -> ()
            n584 = global write "Global Var.vi" "Theta_set"(w510) -> ()
            n585 = global write "Global Var.vi" "Mode PID"(TRUE ("Mode PID")) -> ()
            n586 = global write "Global Var.vi" "ENA"(TRUE ("ENA")) -> ()
            n587 = global write "Global Var.vi" "X_set"(w510) -> ()
            n588 = global write "Global Var.vi" "Y_set"(w510) -> ()
            n589 = global write "Global Var.vi" "Reset"(TRUE ("ENA")) -> ()
            n590 = global write "Global Var.vi" "Speed Low"(FALSE ("Mode PID")) -> ()
            n591 = global write "Global Var.vi" "Vision Mode"(i16 0 ("Vision Mode")) -> ()
            n592 = global write "Global Var.vi" "Servo Kick 2"(u8 255 ("Servo Camera")) -> ()
            n593 = global write "Global Var.vi" "QRCodeTick"(FALSE ("Mode PID")) -> ()
            n594 = global write "Global Var.vi" "Motor_slide1"(FALSE ("Mode PID")) -> ()
            n595 = global write "Global Var.vi" "Motor_rotate"(FALSE ("ENA")) -> ()
            n596 = global write "Global Var.vi" "LED camera"(TRUE ("LED camera")) -> ()
            n597 = global write "Global Var.vi" "Motor_slide2"(FALSE ("ENA")) -> ()
            n598 = global write "Global Var.vi" "Stock"(i16 0 ("Stock")) -> ()
            n599 = global write "Global Var.vi" "BlueBox"(i16 7 ("BlueBox")) -> ()
            n600 = global write "Global Var.vi" "BlueBox (red)"(i16 4 ("BlueBox")) -> ()
            n601 = global write "Global Var.vi" "BlueBox (blue)"(i16 2 ("BlueBox")) -> ()
            n602 = global write "Global Var.vi" "BlueBox (yellow)"(i16 1 ("BlueBox")) -> ()
            n603 = global write "Global Var.vi" "Servo Arm Kick"(u8 70 ("Servo Camera")) -> ()
            n604 = global write "Global Var.vi" "Servo Camera"(u8 134 ("Servo Camera")) -> ()
            n605 = global write "Global Var.vi" "Status"("รอกดสวิตซ์เริ่ม" ("Status")) -> ()
            n606 = global write "Global Var.vi" "Color Box"(u32 6618880 ("Color Box")) -> ()
            n607 = global write "Global Var.vi" "RedBox (yellow)"(i16 1 ("BlueBox")) -> ()
            n608 = global write "Global Var.vi" "RedBox"(i16 7 ("RedBox")) -> ()
            n609 = global write "Global Var.vi" "RedBox (blue)"(i16 4 ("BlueBox")) -> ()
            n610 = global write "Global Var.vi" "RedBox (red)"(i16 2 ("BlueBox")) -> ()
            n611 = global read "Global Var.vi" "Start_SW"() -> (w504:bool)
            n612 = Select(t=101, s=w504, f=100) -> (s? t:f=w485:i32)
          }
          frame 101 {
            n613 = disable-structure shown="Enabled" {
              disable-tunnel: [u32 7821823 ("Color Box") _] -> _
              frame Disabled {
                n614 = call "Step1to2.vi"() -> ()  [unwired: 12 in]
              }
              frame Enabled {
              }
            }
            n615 = call "TEST Blue to Green.vi"() -> ()  [unwired: 12 in]
          }
          frame 102 {
          }
          frame 103 {
            n616 = global write "Global Var.vi" "Status"("ตรวจสอบจำนวนลูก" ("Status")) -> ()
          }
          frame 104 {
            n617 = global write "Global Var.vi" "Status"("Blue to Yellow p1" ("Status")) -> ()
            n618 = call "Blue to yellow 1.vi"() -> ()  [unwired: 12 in]
            n619 = global write "Global Var.vi" "Color Box"(u32 16776722 ("Color Box")) -> ()
            n620 = global write "Global Var.vi" "Yellow No"("2" ("Yellow No")) -> ()
          }
          frame 105 {
            n621 = call "Blue to yellow 2.vi"() -> ()  [unwired: 12 in]
            n622 = global write "Global Var.vi" "Status"("Blue to Yellow p2" ("Status")) -> ()
            n623 = global write "Global Var.vi" "Color Box"(u32 16776722 ("Color Box")) -> ()
            n624 = global write "Global Var.vi" "Yellow No"("2" ("Yellow No")) -> ()
          }
          frame 106 {
            n625 = global write "Global Var.vi" "Status"("Blue to Yellow p3" ("Status")) -> ()
            n626 = call "Blue to yellow 3.vi"() -> ()  [unwired: 12 in]
            n627 = global write "Global Var.vi" "Color Box"(u32 16776722 ("Color Box")) -> ()
            n628 = global write "Global Var.vi" "Yellow No"("2" ("Yellow No")) -> ()
          }
          frame 107 {
            # "วางสีเหลือง Zone  Blue"
            n629 = call "Yellow Place Blue.vi"() -> ()  [unwired: 12 in]
            n630 = global write "Global Var.vi" "Status"("yellow place blue" ("Status")) -> ()
            n631 = global write "Global Var.vi" "Color Box"(u32 16776722 ("Color Box")) -> ()
            n632 = global read "Global Var.vi" "Place 1"() -> (w550:dbl)
            n633 = global read "Global Var.vi" "Place 2"() -> (w548:dbl)
            n634 = global read "Global Var.vi" "Place 3"() -> (w546:dbl)
            n635 = Equal?(x=w550, y=2.0) -> (x = y?=w544:bool)
            n636 = Equal?(x=w548, y=2.0) -> (x = y?=w540:bool)
            n637 = Equal?(x=w546, y=2.0) -> (x = y?=w537:bool)
            n638 = Select(t=110, s=w537, f=1) -> (s? t:f=w538:i32)
            n639 = Select(t=109, s=w540, f=w538) -> (s? t:f=w541:i32)
            n640 = Select(t=108, s=w544, f=w541) -> (s? t:f=w535:i32)
          }
          frame 108 {
            n641 = call "Yellow 1 to blue.vi"() -> ()  [unwired: 12 in]
            n642 = global write "Global Var.vi" "Status"(" yellow p1 to blue" ("Status")) -> ()
          }
          frame 109 {
            n643 = global write "Global Var.vi" "Status"(" yellow p2 to blue" ("Status")) -> ()
            n644 = call "Yellow 2 to blue.vi"() -> ()  [unwired: 12 in]
          }
          frame 110 {
            n645 = global write "Global Var.vi" "Status"(" yellow p3 to blue" ("Status")) -> ()
            n646 = call "Yellow 3 to blue.vi"() -> ()  [unwired: 12 in]
          }
          frame 111 {
            n647 = call "ZoneBlue to ZoneRed.vi"() -> ()  [unwired: 12 in]
          }
          frame 112 {
            # "113"
            n648 = call "ZoneRed rotatePlace.vi"() -> ()  [unwired: 12 in]
            n649 = global write "Global Var.vi" "Status"("ปล่อยลูก Red" ("Status")) -> ()
          }
          frame 113 {
            n650 = flat-sequence {
              frame #0 {
                n651 = call "ZoneRed to Green.vi"() -> ()  [unwired: 12 in]
              }
              frame #1 {
                n652 = local read "lasttime"() -> (w564:u32)
                n653 = local read "time"() -> (w565:u32)
                n654 = Subtract(x=w565, y=w564) -> (x-y=w563:u32)
                n655 = local write "Suctime"(w563) -> ()
                n656 = local write "Reset"(TRUE ("Reset")) -> ()
                n657 = global write "Global Var.vi" "Time"(w563) -> ()
              }
            }
          }
          frame 114 {
            w589 = 0.0 ("X_set")
            n658 = global write "Global Var.vi" "Servo Gripper"(u8 110 ("Servo Camera")) -> ()
            n659 = global write "Global Var.vi" "Servo Kick"(u8 200 ("Servo Camera")) -> ()
            n660 = global write "Global Var.vi" "Servo socket"(u8 150 ("Servo Camera")) -> ()
            n661 = global write "Global Var.vi" "Theta_set"(w589) -> ()
            n662 = global write "Global Var.vi" "Mode PID"(TRUE ("Mode PID")) -> ()
            n663 = global write "Global Var.vi" "ENA"(TRUE ("ENA")) -> ()
            n664 = global write "Global Var.vi" "X_set"(w589) -> ()
            n665 = global write "Global Var.vi" "Y_set"(w589) -> ()
            n666 = global write "Global Var.vi" "Reset"(TRUE ("ENA")) -> ()
            n667 = global write "Global Var.vi" "Speed Low"(FALSE ("Mode PID")) -> ()
            n668 = global write "Global Var.vi" "Servo Kick 2"(u8 255 ("Servo Camera")) -> ()
            n669 = global write "Global Var.vi" "Vision Mode"(i16 0 ("Vision Mode")) -> ()
            n670 = global write "Global Var.vi" "QRCodeTick"(FALSE ("Mode PID")) -> ()
            n671 = global write "Global Var.vi" "Motor_slide1"(FALSE ("Mode PID")) -> ()
            n672 = global write "Global Var.vi" "Motor_rotate"(FALSE ("ENA")) -> ()
            n673 = global write "Global Var.vi" "LED camera"(TRUE ("LED camera")) -> ()
            n674 = global write "Global Var.vi" "Motor_slide2"(FALSE ("ENA")) -> ()
            n675 = global write "Global Var.vi" "Stock"(i16 0 ("Stock")) -> ()
            n676 = global write "Global Var.vi" "BlueBox"(i16 7 ("BlueBox")) -> ()
            n677 = global write "Global Var.vi" "BlueBox (red)"(i16 4 ("BlueBox")) -> ()
            n678 = global write "Global Var.vi" "BlueBox (blue)"(i16 2 ("BlueBox")) -> ()
            n679 = global write "Global Var.vi" "BlueBox (yellow)"(i16 1 ("BlueBox")) -> ()
            n680 = global write "Global Var.vi" "Status"("รอกดสวิตซ์เริ่ม" ("Status")) -> ()
            n681 = global write "Global Var.vi" "Color Box"(u32 6618880 ("Color Box")) -> ()
            n682 = global write "Global Var.vi" "RedBox (yellow)"(i16 1 ("BlueBox")) -> ()
            n683 = global write "Global Var.vi" "RedBox"(i16 7 ("RedBox")) -> ()
            n684 = global write "Global Var.vi" "RedBox (blue)"(i16 4 ("BlueBox")) -> ()
            n685 = global write "Global Var.vi" "RedBox (red)"(i16 2 ("BlueBox")) -> ()
            n686 = global read "Global Var.vi" "Start_SW"() -> (w584:bool)
            n687 = Select(t=115, s=w584, f=114) -> (s? t:f=w566:i32)
          }
          frame 115 {
            n688 = call "TEST Blue to Green.vi"() -> ()  [unwired: 12 in]
            n689 = disable-structure shown="Disabled" {
              frame Disabled {
              }
              frame Enabled {
              }
            }
          }
          frame 200 {
            w623 = 0.0 ("X_set")
            n690 = global write "Global Var.vi" "Servo Gripper"(u8 110 ("Servo Camera")) -> ()
            n691 = global write "Global Var.vi" "Servo Kick"(u8 200 ("Servo Camera")) -> ()
            n692 = global write "Global Var.vi" "Servo socket"(u8 150 ("Servo Camera")) -> ()
            n693 = global write "Global Var.vi" "Theta_set"(w623) -> ()
            n694 = global write "Global Var.vi" "Mode PID"(TRUE ("Mode PID")) -> ()
            n695 = global write "Global Var.vi" "ENA"(TRUE ("ENA")) -> ()
            n696 = global write "Global Var.vi" "X_set"(w623) -> ()
            n697 = global write "Global Var.vi" "Y_set"(w623) -> ()
            n698 = global write "Global Var.vi" "Reset"(TRUE ("ENA")) -> ()
            n699 = global write "Global Var.vi" "Speed Low"(FALSE ("Mode PID")) -> ()
            n700 = global write "Global Var.vi" "Servo Kick 2"(u8 255 ("Servo Camera")) -> ()
            n701 = global write "Global Var.vi" "Vision Mode"(i16 0 ("Vision Mode")) -> ()
            n702 = global write "Global Var.vi" "QRCodeTick"(FALSE ("Mode PID")) -> ()
            n703 = global write "Global Var.vi" "Motor_slide1"(FALSE ("Mode PID")) -> ()
            n704 = global write "Global Var.vi" "Motor_rotate"(FALSE ("ENA")) -> ()
            n705 = global write "Global Var.vi" "LED camera"(TRUE ("LED camera")) -> ()
            n706 = global write "Global Var.vi" "Motor_slide2"(FALSE ("ENA")) -> ()
            n707 = global write "Global Var.vi" "Stock"(i16 0 ("Stock")) -> ()
            n708 = global write "Global Var.vi" "BlueBox"(i16 7 ("BlueBox")) -> ()
            n709 = global write "Global Var.vi" "BlueBox (red)"(i16 4 ("BlueBox")) -> ()
            n710 = global write "Global Var.vi" "BlueBox (blue)"(i16 2 ("BlueBox")) -> ()
            n711 = global write "Global Var.vi" "BlueBox (yellow)"(i16 1 ("BlueBox")) -> ()
            n712 = global write "Global Var.vi" "Servo_Arm_Kick_main"(FALSE ("Mode PID")) -> ()
            n713 = global write "Global Var.vi" "Servo_Camera_main"(FALSE ("Mode PID")) -> ()
            n714 = global write "Global Var.vi" "Line Dis X"(TRUE ("Mode PID")) -> ()
            n715 = global write "Global Var.vi" "Status"("รอกดสวิตซ์เริ่ม" ("Status")) -> ()
            n716 = global write "Global Var.vi" "Color Box"(u32 6618880 ("Color Box")) -> ()
            n717 = global write "Global Var.vi" "RedBox (yellow)"(i16 1 ("BlueBox")) -> ()
            n718 = global write "Global Var.vi" "RedBox"(i16 7 ("RedBox")) -> ()
            n719 = global write "Global Var.vi" "RedBox (blue)"(i16 4 ("BlueBox")) -> ()
            n720 = global write "Global Var.vi" "RedBox (red)"(i16 2 ("BlueBox")) -> ()
            n721 = global read "Global Var.vi" "Start_SW"() -> (w618:bool)
            n722 = disable-structure shown="Disabled" {
              frame Disabled {
                n723 = global write "Global Var.vi" "Place 1"(2.0 ("Place 3")) -> ()
                n724 = global write "Global Var.vi" "Place 2"(1.0 ("Place 3")) -> ()
                n725 = global write "Global Var.vi" "Place 3"(3.0 ("Place 3")) -> ()
              }
              frame Enabled {
              }
            }
            n726 = Select(t=201, s=w618, f=200) -> (s? t:f=w600:i32)
          }
          frame 201 {
            n727 = disable-structure shown="Enabled" {
              frame Enabled {
                n728 = flat-sequence {
                  frame #0 {
                    n729 = call "TEST Blue to Green.vi"() -> ()  [unwired: 12 in]
                  }
                  frame #1 {
                    n730 = call "ZoneRed to ZoneBlue.vi"() -> ()  [unwired: 12 in]
                  }
                }
              }
              frame Disabled {
              }
            }
            n731 = disable-structure shown="Disabled" {
              frame Disabled {
                n732 = call "TEST Blue to Green.vi"() -> ()  [unwired: 12 in]
              }
              frame Enabled {
              }
            }
          }
          frame 205 {
            w659 = 0.0 ("X_set")
            n733 = global write "Global Var.vi" "Servo Gripper"(u8 110 ("Servo Camera")) -> ()
            n734 = global write "Global Var.vi" "Servo Kick"(u8 200 ("Servo Camera")) -> ()
            n735 = global write "Global Var.vi" "Servo socket"(u8 150 ("Servo Camera")) -> ()
            n736 = global write "Global Var.vi" "Theta_set"(w659) -> ()
            n737 = global write "Global Var.vi" "Mode PID"(TRUE ("Mode PID")) -> ()
            n738 = global write "Global Var.vi" "ENA"(TRUE ("ENA")) -> ()
            n739 = global write "Global Var.vi" "X_set"(w659) -> ()
            n740 = global write "Global Var.vi" "Y_set"(w659) -> ()
            n741 = global write "Global Var.vi" "Reset"(TRUE ("ENA")) -> ()
            n742 = global write "Global Var.vi" "Speed Low"(FALSE ("Mode PID")) -> ()
            n743 = global write "Global Var.vi" "Servo Kick 2"(u8 255 ("Servo Camera")) -> ()
            n744 = global write "Global Var.vi" "Vision Mode"(i16 0 ("Vision Mode")) -> ()
            n745 = global write "Global Var.vi" "QRCodeTick"(FALSE ("Mode PID")) -> ()
            n746 = global write "Global Var.vi" "Motor_slide1"(FALSE ("Mode PID")) -> ()
            n747 = global write "Global Var.vi" "Motor_rotate"(FALSE ("ENA")) -> ()
            n748 = global write "Global Var.vi" "LED camera"(TRUE ("LED camera")) -> ()
            n749 = global write "Global Var.vi" "Motor_slide2"(FALSE ("ENA")) -> ()
            n750 = global write "Global Var.vi" "Stock"(i16 0 ("Stock")) -> ()
            n751 = global write "Global Var.vi" "BlueBox"(i16 7 ("BlueBox")) -> ()
            n752 = global write "Global Var.vi" "BlueBox (red)"(i16 4 ("BlueBox")) -> ()
            n753 = global write "Global Var.vi" "BlueBox (blue)"(i16 2 ("BlueBox")) -> ()
            n754 = global write "Global Var.vi" "BlueBox (yellow)"(i16 1 ("BlueBox")) -> ()
            n755 = global write "Global Var.vi" "Servo_Arm_Kick_main"(FALSE ("Mode PID")) -> ()
            n756 = global write "Global Var.vi" "Servo_Camera_main"(FALSE ("Mode PID")) -> ()
            n757 = global write "Global Var.vi" "Status"("รอกดสวิตซ์เริ่ม" ("Status")) -> ()
            n758 = global write "Global Var.vi" "Color Box"(u32 6618880 ("Color Box")) -> ()
            n759 = global write "Global Var.vi" "RedBox (yellow)"(i16 1 ("BlueBox")) -> ()
            n760 = global write "Global Var.vi" "RedBox"(i16 7 ("RedBox")) -> ()
            n761 = global write "Global Var.vi" "RedBox (blue)"(i16 4 ("BlueBox")) -> ()
            n762 = global write "Global Var.vi" "RedBox (red)"(i16 2 ("BlueBox")) -> ()
            n763 = global read "Global Var.vi" "Start_SW"() -> (w654:bool)
            n764 = Select(t=206, s=w654, f=205) -> (s? t:f=w636:i32)
          }
          frame 206 {
            n765 = flat-sequence {
              frame #0 {
                n766 = call "TEST Blue to Green.vi"() -> ()  [unwired: 12 in]
              }
              frame #1 {
                n767 = call "ZoneBlue to ZoneRed.vi"() -> ()  [unwired: 12 in]
              }
            }
          }
          frame 210 {
            w692 = 0.0 ("X_set")
            n768 = global write "Global Var.vi" "Servo Gripper"(u8 110 ("Servo Camera")) -> ()
            n769 = global write "Global Var.vi" "Servo Kick"(u8 200 ("Servo Camera")) -> ()
            n770 = global write "Global Var.vi" "Servo socket"(u8 150 ("Servo Camera")) -> ()
            n771 = global write "Global Var.vi" "Theta_set"(w692) -> ()
            n772 = global write "Global Var.vi" "Mode PID"(TRUE ("Mode PID")) -> ()
            n773 = global write "Global Var.vi" "ENA"(TRUE ("ENA")) -> ()
            n774 = global write "Global Var.vi" "X_set"(w692) -> ()
            n775 = global write "Global Var.vi" "Y_set"(w692) -> ()
            n776 = global write "Global Var.vi" "Reset"(TRUE ("ENA")) -> ()
            n777 = global write "Global Var.vi" "Speed Low"(FALSE ("Mode PID")) -> ()
            n778 = global write "Global Var.vi" "Servo Kick 2"(u8 255 ("Servo Camera")) -> ()
            n779 = global write "Global Var.vi" "Vision Mode"(i16 0 ("Vision Mode")) -> ()
            n780 = global write "Global Var.vi" "QRCodeTick"(FALSE ("Mode PID")) -> ()
            n781 = global write "Global Var.vi" "Motor_slide1"(FALSE ("Mode PID")) -> ()
            n782 = global write "Global Var.vi" "Motor_rotate"(FALSE ("ENA")) -> ()
            n783 = global write "Global Var.vi" "LED camera"(TRUE ("LED camera")) -> ()
            n784 = global write "Global Var.vi" "Motor_slide2"(FALSE ("ENA")) -> ()
            n785 = global write "Global Var.vi" "Stock"(i16 0 ("Stock")) -> ()
            n786 = global write "Global Var.vi" "BlueBox"(i16 7 ("BlueBox")) -> ()
            n787 = global write "Global Var.vi" "BlueBox (red)"(i16 4 ("BlueBox")) -> ()
            n788 = global write "Global Var.vi" "BlueBox (blue)"(i16 2 ("BlueBox")) -> ()
            n789 = global write "Global Var.vi" "BlueBox (yellow)"(i16 1 ("BlueBox")) -> ()
            n790 = global write "Global Var.vi" "Servo_Arm_Kick_main"(TRUE ("Mode PID")) -> ()
            n791 = global write "Global Var.vi" "Servo_Camera_main"(FALSE ("Mode PID")) -> ()
            n792 = global write "Global Var.vi" "Status"("รอกดสวิตซ์เริ่ม" ("Status")) -> ()
            n793 = global write "Global Var.vi" "Color Box"(u32 6618880 ("Color Box")) -> ()
            n794 = global write "Global Var.vi" "RedBox (yellow)"(i16 1 ("BlueBox")) -> ()
            n795 = global write "Global Var.vi" "RedBox"(i16 7 ("RedBox")) -> ()
            n796 = global write "Global Var.vi" "RedBox (blue)"(i16 4 ("BlueBox")) -> ()
            n797 = global write "Global Var.vi" "RedBox (red)"(i16 2 ("BlueBox")) -> ()
            n798 = global read "Global Var.vi" "Start_SW"() -> (w687:bool)
            n799 = Select(t=211, s=w687, f=210) -> (s? t:f=w669:i32)
          }
          frame 211 {
            n800 = call "find_position.vi"() -> ()  [unwired: 12 in]
          }
        }
        n801 = Wait (ms)(milliseconds to wait=u32 10) -> ()  [unwired: 1 out]
      }
      n802 = while {
        stop <- w78 stop-if-true
        n803 = global read "Global Var.vi" "Stop"() -> (w78:bool)
        n804 = global read "Global Var.vi" "Stop"() -> (w77:bool)
        n805 = call "Vision Acquisition"("Stop (F)"=w77) -> ("Image Out"=w75:T14)  [unwired: 24 in, 2 out]
        n806 = global read "Global Var.vi" "Vision Mode"() -> (w76:i16)
        n807 = Wait (ms)(milliseconds to wait=u32 10) -> ()  [unwired: 1 out]
        n808 = case shown="6" w76 {
          tunnel: w75 -> [w80 w88 w90 w99 w108 w124 w137]
          frame 0, Default {
            n809 = global write "Global Var.vi" "Image_line"(w80) -> ()
          }
          frame 3 {
            n810 = call "Vision Assistant"("Image In"=w88) -> ("Image Out"=w89:T14, "Straight Edge (Find Straight Edge 1)"=w87:T15, "Straight Edge (Find Straight Edge 2)"=w86:T15)  [unwired: 23 in, 1 out]
            n811 = disable-structure shown="Disabled" {
              frame Disabled {
              }
              frame Enabled {
              }
            }
            n812 = Unbundle By Name(w87) -> ("Point1 (Pixels)"=w85:cluster{"X":sgl, "Y":sgl}, "Angle (Pixel)"=w82:dbl)
            n813 = Unbundle By Name(w86) -> ("Point1 (Pixels)"=w84:cluster{"X":sgl, "Y":sgl})
            n814 = Unbundle(w84) -> ("Y"=w83:sgl)  [unwired: 1 out]
            n815 = Unbundle(w85) -> ("X"=w81:sgl)  [unwired: 1 out]
            n816 = global write "Global Var.vi" "Image_line"(w89) -> ()
            n817 = global write "Global Var.vi" "Cross Line Position"(w83) -> ()
            n818 = global write "Global Var.vi" "X_Line"(w81) -> ()
            n819 = global write "Global Var.vi" "Angle_Line"(w82) -> ()
          }
          frame 4 {
            # "Red"
            n820 = call "Vision Assistant3"("Image In"=w90) -> ("Image Out"=w98:T14, "Straight Edges (Adv. Straight Edge 1)"=w97:T16, "Straight Edges (Adv. Straight Edge 3)"=w94:T16)  [unwired: 23 in, 1 out]
            n821 = Array To Cluster(array=w97) -> (cluster=w96:T17)
            n822 = Array To Cluster(array=w94) -> (cluster=w93:T18)
            n823 = Unbundle By Name(w96) -> ("Straight Edges (Adv. Straight Edge 1)[0].Point1 (Pixels).X"=w92:sgl, "Straight Edges (Adv. Straight Edge 1)[0].Angle (Pixel)"=w95:dbl)
            n824 = Unbundle By Name(w93) -> ("Straight Edges (Adv. Straight Edge 3)[0].Point1 (Pixels).Y"=w91:sgl)
            n825 = global write "Global Var.vi" "Cross Line Position"(w91) -> ()
            n826 = global write "Global Var.vi" "X_Line"(w92) -> ()
            n827 = global write "Global Var.vi" "Angle_Line"(w95) -> ()
            n828 = global write "Global Var.vi" "Image_line"(w98) -> ()
          }
          frame 5 {
            # "Yellow"
            n829 = call "Vision Assistant4"("Image In"=w99) -> ("Image Out"=w107:T14, "Straight Edges (Adv. Straight Edge 1)"=w106:T16, "Straight Edges (Adv. Straight Edge 3)"=w103:T16)  [unwired: 23 in, 1 out]
            n830 = Array To Cluster(array=w106) -> (cluster=w105:T17)
            n831 = Array To Cluster(array=w103) -> (cluster=w102:T18)
            n832 = Unbundle By Name(w105) -> ("Straight Edges (Adv. Straight Edge 1)[0].Point1 (Pixels).X"=w101:sgl, "Straight Edges (Adv. Straight Edge 1)[0].Angle (Pixel)"=w104:dbl)
            n833 = Unbundle By Name(w102) -> ("Straight Edges (Adv. Straight Edge 3)[0].Point1 (Pixels).Y"=w100:sgl)
            n834 = global write "Global Var.vi" "Cross Line Position"(w100) -> ()
            n835 = global write "Global Var.vi" "X_Line"(w101) -> ()
            n836 = global write "Global Var.vi" "Angle_Line"(w104) -> ()
            n837 = global write "Global Var.vi" "Image_line"(w107) -> ()
          }
          frame 6 {
            # "may be blue sometime"
            # "White"
            n838 = call "Vision Assistant5"("Image In"=w108) -> ("Image Out"=w109:T14, "Straight Edges (Adv. Straight Edge 1)"=w110:T16, "Straight Edges (Adv. Straight Edge 3)"=w113:T16)  [unwired: 23 in, 1 out]
            n839 = Array To Cluster(array=w110) -> (cluster=w111:T17)
            n840 = Array To Cluster(array=w113) -> (cluster=w114:T18)
            n841 = Unbundle By Name(w111) -> ("Straight Edges (Adv. Straight Edge 1)[0].Point1 (Pixels).X"=w115:sgl, "Straight Edges (Adv. Straight Edge 1)[0].Angle (Pixel)"=w112:dbl)
            n842 = Unbundle By Name(w114) -> ("Straight Edges (Adv. Straight Edge 3)[0].Point1 (Pixels).Y"=w116:sgl)
            n843 = global write "Global Var.vi" "Cross Line Position"(w116) -> ()
            n844 = global write "Global Var.vi" "X_Line"(w115) -> ()
            n845 = global write "Global Var.vi" "Angle_Line"(w112) -> ()
            n846 = global write "Global Var.vi" "Image_line"(w109) -> ()
          }
          frame 2 {
            n847 = call "Vision Yellow"("Image In"=w124) -> ("Image Out"=w123:T14, "Number of Matches (Color Location 1)"=w118:i32)  [unwired: 24 in, 1 out]
            n848 = call "Vision Blue"("Image In"=w124) -> ("Image Out"=w130:T14, "Number of Matches (Color Location 1)"=w131:i32)  [unwired: 24 in, 1 out]
            n849 = call "Vision Red"("Image In"=w124) -> ("Image Out"=w126:T14, "Number of Matches (Color Location 1)"=w125:i32)  [unwired: 24 in, 1 out]
            n850 = global write "Global Var.vi" "Image_line"(w123) -> ()
            n851 = global write "Global Var.vi" "Image_line"(w126) -> ()
            n852 = global write "Global Var.vi" "Image_line"(w130) -> ()
            n853 = Equal?(x=w131, y=1) -> (x = y?=w134:bool)
            n854 = Select(t="Blue", s=w134, f="No Color") -> (s? t:f=w136:string)
            n855 = Equal?(x=w125, y=1) -> (x = y?=w128:bool)
            n856 = Select(t="Red", s=w128, f=w136) -> (s? t:f=w119:string)
            n857 = Equal?(x=w118, y=1) -> (x = y?=w121:bool)
            n858 = Select(t="Yellow", s=w121, f=w119) -> (s? t:f=w117:string)
            n859 = global write "Global Var.vi" "Color"(w117) -> ()
          }
          frame 1 {
            # "Blue"
            n860 = call "Vision Assistant2"("Image In"=w137) -> ("Image Out"=w145:T14, "Straight Edges (Adv. Straight Edge 1)"=w144:T16, "Straight Edges (Adv. Straight Edge 3)"=w141:T16)  [unwired: 23 in, 1 out]
            n861 = Array To Cluster(array=w144) -> (cluster=w143:T17)
            n862 = Array To Cluster(array=w141) -> (cluster=w140:T18)
            n863 = Unbundle By Name(w143) -> ("Straight Edges (Adv. Straight Edge 1)[0].Point1 (Pixels).X"=w139:sgl, "Straight Edges (Adv. Straight Edge 1)[0].Angle (Pixel)"=w142:dbl)
            n864 = Unbundle By Name(w140) -> ("Straight Edges (Adv. Straight Edge 3)[0].Point1 (Pixels).Y"=w138:sgl)
            n865 = global write "Global Var.vi" "Cross Line Position"(w138) -> ()
            n866 = global write "Global Var.vi" "X_Line"(w139) -> ()
            n867 = global write "Global Var.vi" "Angle_Line"(w142) -> ()
            n868 = global write "Global Var.vi" "Image_line"(w145) -> ()
          }
        }
      }
      n869 = while {
        stop <- w74 stop-if-true
        n870 = call "Elapsed Time"("Reset"="Reset", "Set Start Time (s)"=0.0) -> ("Elapsed Time (s)"=→"time":dbl)  [unwired: 10 in, 7 out]
        n871 = global read "Global Var.vi" "Stop"() -> (w74:bool)
      }
    }
    frame #2 {
      w1208 = i16 0 ("INSpeed 1")
      w1209 = 0.0 ("X_set")
      n872 = disable-structure shown="Disabled" {
        frame Disabled {
          # "Yellow"
          # "Blue"
          # "RED"
          n873 = global write "Global Var.vi" "Vision Mode"(i16 6 ("Vision Mode")) -> ()
          n874 = global write "Global Var.vi" "Vision Mode"(i16 4 ("Vision Mode")) -> ()
          n875 = global write "Global Var.vi" "Vision Mode"(i16 5 ("Vision Mode")) -> ()
        }
        frame Enabled {
        }
      }
      n876 = global write "Global Var.vi" "Servo Camera"(u8 200 ("Servo Camera")) -> ()
      n877 = global write "Global Var.vi" "Servo Gripper"(u8 110 ("Servo Camera")) -> ()
      n878 = global write "Global Var.vi" "Servo Kick"(u8 200 ("Servo Camera")) -> ()
      n879 = global write "Global Var.vi" "Servo Arm Kick"(u8 165 ("Servo Camera")) -> ()
      n880 = global write "Global Var.vi" "Servo socket"(u8 100 ("Servo Camera")) -> ()
      n881 = global write "Global Var.vi" "INSpeed 1"(w1208) -> ()
      n882 = global write "Global Var.vi" "INSpeed 2"(w1208) -> ()
      n883 = global write "Global Var.vi" "INSpeed 3"(w1208) -> ()
      n884 = global write "Global Var.vi" "Servo Kick 2"(u8 255 ("Servo Camera")) -> ()
      n885 = global write "Global Var.vi" "Mode PID"(TRUE ("Mode PID")) -> ()
      n886 = global write "Global Var.vi" "ENA"(TRUE ("ENA")) -> ()
      n887 = global write "Global Var.vi" "Reset"(TRUE ("ENA")) -> ()
      n888 = global write "Global Var.vi" "Line Dis"(FALSE ("Mode PID")) -> ()
      n889 = VISA Close(VISA resource name=w1203, error in (no error)=w1204) -> ()  [unwired: 1 out]
      n890 = VISA Close(VISA resource name=w1206, error in (no error)=w1205) -> ()  [unwired: 1 out]
      n891 = global write "Global Var.vi" "Motor_slide1"(FALSE ("ENA")) -> ()
      n892 = global write "Global Var.vi" "Motor_rotate"(FALSE ("ENA")) -> ()
      n893 = global write "Global Var.vi" "Theta_set"(w1209) -> ()
      n894 = global write "Global Var.vi" "LED camera"(TRUE ("Mode PID")) -> ()
      n895 = global write "Global Var.vi" "X_set"(w1209) -> ()
      n896 = global write "Global Var.vi" "Y_set"(w1209) -> ()
      n897 = global write "Global Var.vi" "Motor_slide2"(FALSE ("LED camera")) -> ()
    }
  }
  n898 = global write "Global Var.vi" "Servo Camera"(u8 200 ("Servo Camera")) -> ()
  n899 = global write "Global Var.vi" "Servo Gripper"(u8 110 ("Servo Camera")) -> ()
  n900 = global write "Global Var.vi" "Servo Kick"(u8 200 ("Servo Camera")) -> ()
  n901 = global write "Global Var.vi" "Servo Arm Kick"(u8 165 ("Servo Camera")) -> ()
  n902 = global write "Global Var.vi" "Servo socket"(u8 100 ("Servo Camera")) -> ()
  n903 = global write "Global Var.vi" "Servo Kick 2"(u8 255 ("Servo Camera")) -> ()
  n904 = global write "Global Var.vi" "INSpeed 1"(w10) -> ()
  n905 = global write "Global Var.vi" "INSpeed 2"(w10) -> ()
  n906 = global write "Global Var.vi" "INSpeed 3"(w10) -> ()
  n907 = global write "Global Var.vi" "Mode PID"(TRUE ("Mode PID")) -> ()
  n908 = global write "Global Var.vi" "ENA"(TRUE ("ENA")) -> ()
  n909 = global write "Global Var.vi" "Reset"(TRUE ("ENA")) -> ()
  n910 = global write "Global Var.vi" "Line Dis"(FALSE ("Mode PID")) -> ()
  n911 = global write "Global Var.vi" "Motor_slide1"(FALSE ("ENA")) -> ()
  n912 = global write "Global Var.vi" "Motor_rotate"(FALSE ("ENA")) -> ()
  n913 = global write "Global Var.vi" "Theta_set"(w11) -> ()
  n914 = global write "Global Var.vi" "LED camera"(TRUE ("Mode PID")) -> ()
  n915 = global write "Global Var.vi" "X_set"(w11) -> ()
  n916 = global write "Global Var.vi" "Y_set"(w11) -> ()
  n917 = global write "Global Var.vi" "Motor_slide2"(FALSE ("LED camera")) -> ()
  n918 = disable-structure shown="Disabled" {
    frame Disabled {
      # "มุมเตะ"
      # "True"
      # "False"
      # "เก็บServo"
      # "มุมตั้งตรง"
      # "มุม Track line"
      n919 = global write "Global Var.vi" "Servo Arm Kick"(u8 70 ("Servo Camera")) -> ()
      n920 = global write "Global Var.vi" "Servo Camera"(u8 200 ("Servo Camera")) -> ()
      n921 = global write "Global Var.vi" "Servo Camera"(u8 134 ("Servo Camera")) -> ()
      n922 = global write "Global Var.vi" "Servo Arm Kick"(u8 165 ("Servo Camera")) -> ()
    }
    frame Enabled {
    }
  }
